vi "DigData.vi"(0 "Type of scan":T14, 1 "Digitizer Settings":T10={"Digitizer delay (us) "=0.0, "rf points per line"=2048, "lines per plane"=128, "Samp Rate (Hz)"=100000000.0, "Additional dig delay (us)"=0.0, "Voltage Scale"=0.4, "Pre-Looks"=0, "Offset delay (us)"=0.0, "bits A/D"=8, "Avg Num"=1, "DigTimeOut"=5.0, "Rel Dig Delay"=0.0, "Dig Ch"=0, "LeCroyCluster"={"LeCroy Channels"=[TRUE, FALSE, FALSE, FALSE], "LC read pt offset"=0.0, "Sweep Avg"=FALSE}, "Main Digitizer"=enum."NI Digitizer", "Dig Config"=enum."Single channel", "Digitizer ID Cluster"={"Acqiris/Alazar/SP ID"=[], "NI Instr Handles"=[], "LeCroy VISA"="", "GaGe Handle"={"Handle"=0, "Sample size"=0, "Resolution"=0, "Offset"=0, "Channels"=0, "Boards"=0}, "ATS Ref"="ATS9350", "Acqiris Address"=["PCI::INSTR0"], "ADQRef"=refnum, "adq_cu_ptr"=refnum}, "Trigger Settings"={"Trig Source"=1, "Trig Coupling"=0, "Trig Slope"=0, "Level (mV)"=1500.0}, "Bulk Acq"=FALSE, "Bulk Start Indexes"=[], "Data Ref RF"=refnum, "NI ID/Channel"=[], "Total Dig CH"=1, "Xtra Ann Trig delay (us)"=10.0, "Fix Z Delay?"=FALSE, "One Way Transmission?"=FALSE, "Data Ref Log"=refnum} {"Trigger Settings"."Trig Slope" items=["Positive", "Negative"]; "Trigger Settings"."Level (mV)" format="%.2f"; "Trigger Settings"."Trig Coupling" items=["DC 1 MOhm", "AC 1 MOhm", "DC 50 Ohm", "AC 50 Ohm"]; "Trigger Settings"."Trig Source" items=["Chan 1", "External"]; "Rel Dig Delay" format="%.2f"; "DigTimeOut" format="%.2f"; "Avg Num" min=1; "Offset delay (us)" format="%.2f"; "Additional dig delay (us)" format="%.2f"; "Digitizer delay (us)" format="%.2f"}, 5 "File Name In":string, 7 "Therapy (T)":bool, 8 "Ann Array Params":T3={"Synth Foc?"=FALSE, "Focal Zones"=41, "Switch T/R"=0, "Trans Geometry (mm)"={"Transducer"=0, "Geo Focus"=12.0, "a (radius)"=3.0, "# of rings"=5, "kerf space "=0.1, "Center Freq"=12.0}, "Sub Ap Excite?"=FALSE, "Full Array Scan?"=FALSE, "Xmt/Rcv"={"XMIT"=[TRUE, TRUE, TRUE, TRUE, TRUE], "RCV"=[TRUE, TRUE, TRUE, TRUE, TRUE]}, "PulseSpacing (us)"=0.0, "Xmit Ring"=0, "XMIT CHS"=0, "RCV CHS"=0, "GPU?"=FALSE, "Save TIFF?"=FALSE, "downfactor"=1, "RCV 1CH"=0} {"RCV 1CH" items=["All", "1", "2", "3", "4", "5"]; "Trans Geometry (mm)"."Transducer" items=["6D 12R 40 MHz"=0, "10D 31R 20 MHz"=1, "10D 23R 20 MHz"=2, "6D 23R 40 MHz"=3, "4.5D 10.7R 40 MHz"=4, "9D 23.5R 20 MHz"=5, "9D 25.8R 20MHz"=6, "Enter"=99]; "Switch T/R" min=1 max=5 step=1}, 9 "Motion Settings In":T6={"No Motion?"=FALSE, "Motion System"=enum."NI 735x", "Motion Bd ID"=1, "Motion Profile"="SMAC1", "# Axis"=1, "Reverse Z axis?"=TRUE, "SMAC Axis"=0, "scan pair"=enum."y-(x) scan", "RT fps"=6.0, "Steps per mm"=[1000, 1000, 1000, 1000], "Motor Parameters"={"velocity ct/s"=[10000.0, 10000.0, 10000.0, 50000.0], "accel ct/s^2"=[50000.0, 50000.0, 50000.0, 200000.0]}, "One Way Scan"=FALSE, "Reverse One Way Scan"=FALSE, "Global Position (mm)"=[], "Plane"=0, "Distance between\nscan lines (um)"=0.0, "Distance between\nscan planes (um)"=0.0, "number of scan planes"=1, "Total steps in line"=0, "Xtra plane\ndistance  (um)"=100, "Xtra planes "=1, "Add Axis"=FALSE, "overshoot cts"=200, "BKPT Shift"=0, "Scan Start Time (ms)"=0, "ESP VISA"="GPIB::1::INSTR", "3rd Axis"=1, "GL Ref Out"=refnum, "Galil Address"=""} {"3rd Axis" items=["x", "y", "z", "w"]; "Xtra planes" min=1; "Xtra plane\ndistance  (um)" min=0; "Distance between\nscan planes (um)" format="%.2f"; "Distance between\nscan lines (um)" format="%.2f"; "SMAC Axis" items=["None"=0, "Axis 1"=1, "Axis 2"=2, "Axis 3"=3, "Axis 4"=4, "Axis 5"=5, "Axis 6"=6, "Axis 7"=7, "Axis 8"=8, "Vector Space 1"=17, "Vector Space 2"=18, "Vector Space 3"=19, "Vector Space 4"=20]; "Motion Bd ID" min=1 max=32 step=1}, 10 "recipient":string, 11 "Microscopy Scan Mode":T2(ring)=enum."Overview Scan", 12 "Breath Divide":i32=1) -> (20 "Scan Params":T1={"File Name"="", "Keep?"=FALSE, "Synth Foc?"=FALSE, "Microscopy Scan Mode"=enum."Overview Scan"}, 27 "Error Message":string)   [LabVIEW 2022 SP3]
uses:
  Controls/ScanType2.ctl
  Digitizers/-DigitizerRoutines/DigitizerSettings.ctl
  Digitizers/-DigitizerRoutines/Digitizer.ctl
  Digitizers/-DigitizerRoutines/DigConfig.ctl
  Digitizers/-DigitizerRoutines/DigitizerID.ctl
  C:/Windows/System32/ADQAPI_dotNet_helper.dll
  Windows/System32/ADQAPI_dotNet_helper.dll
  Motion Controllers/NI_controller/-NI_MotionRoutines/MotionParameters.ctl
  Motion Controllers/NI_controller/-NI_MotionRoutines/MotionSys.ctl
  Motion Controllers/-MotionRoutines/ScanAxis.ctl
  Motion Controllers/-MotionRoutines/3rdAxis.ctl
  Annular Array/-AnnularRoutines/AnnularArray.ctl
  Annular Array/-AnnularRoutines/TransGeometry.ctl
  Annular Array/-AnnularRoutines/ArrayGeometry.ctl
  Controls/ScanParams.ctl
  Motion Controllers/Galil/Command Menu.ctl
  <vilib>/DAQmx/write.llb/DAQmx Write (Digital Bool 1Line 1Point).vi
  Motion Controllers/-MotionRoutines/MotionGlobals.vi
  Pulsers/PulserGlobals.vi
  <vilib>/DAQmx/create/channels.llb/DAQmx Create Channel (CO-Pulse Generation-Frequency).vi
  <vilib>/DAQmx/configure/timing.llb/DAQmx Timing (Implicit).vi
  <vilib>/DAQmx/miscellaneous.llb/DAQmx Fill In Error Info.vi
  <vilib>/DAQmx/create/channels.llb/DAQmx Create Channel (AI-Voltage-Basic).vi
  <vilib>/DAQmx/configure/timing.llb/DAQmx Timing (Sample Clock).vi
  <vilib>/DAQmx/configure/trigger.llb/DAQmx Start Trigger (Digital Edge).vi
  Switch Modules/SwitchGlobals.vi
  Motion Controllers/Galil/GL Axis Control.ctl
  <vilib>/Utility/SMTP/NI_SMTPEmail.lvlib
  <vilib>/Motion/FlexMotion/CustomControls/CustomControls.llb/Mask (8 axes).flx
  <vilib>/Motion/FlexMotion/FunctionsVIs/Trajectory.llb/Load Acceleration/Deceleration.flx
  <instrlib>/Newport ESP301/Newport ESP301.lvlib
  <instrlib>/LeCroy Wave Series/LeCroy Wave Series.lvlib
  <vilib>/Motion/FlexMotion/FunctionsVIs/MotionIO.llb/Set Inhibit MOMO (8 axes).flx
panel:
  out "x-y":u32
  out "Current Plane":i32
  # "First axis used in 1-D\nscan"
  # "1-D and 2-D B scan settings"
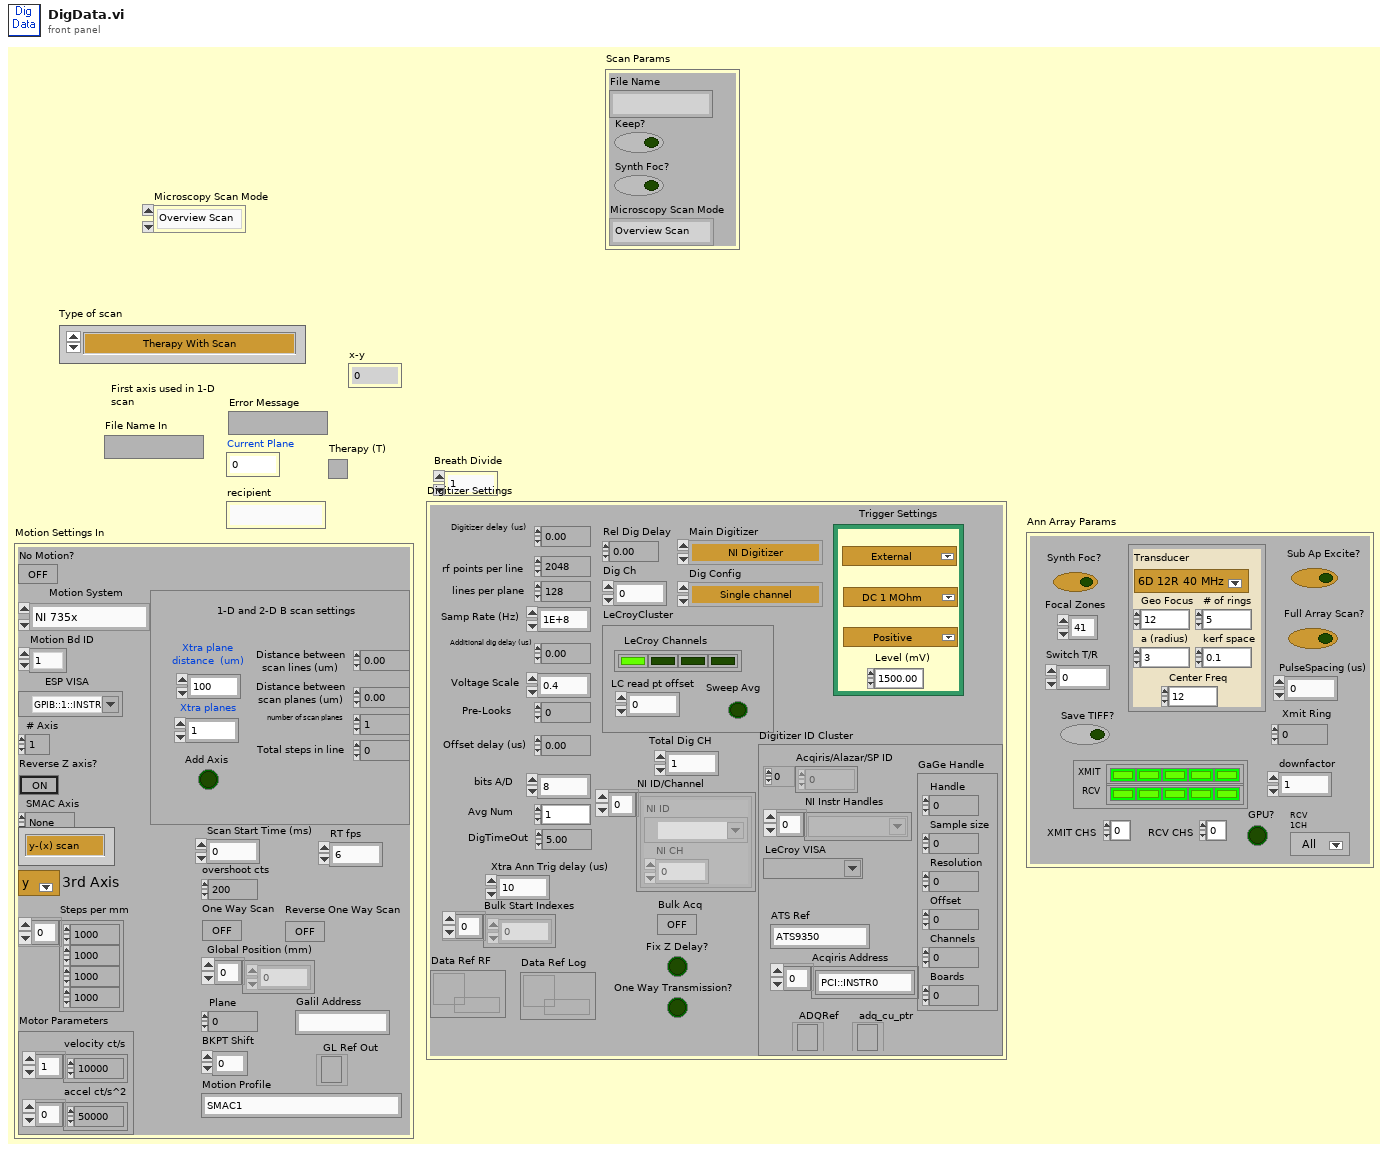
[diagram p1: front panel]
types:
  T1 = typedef "ScanParams.ctl" = cluster{"File Name":string, "Keep?":bool, "Synth Foc?":bool, "Microscopy Scan Mode":enum32{"Level X", "Level Y", "Overview Scan", "Detailed Scan", "V-Z Scan"}}
  T2 = enum32{"Level X", "Level Y", "Overview Scan", "Detailed Scan", "V-Z Scan"}
  T3 = typedef "AnnularArray.ctl" = cluster{"Synth Foc?":bool, "Focal Zones":i16, "Switch T/R":i16, "Trans Geometry (mm)":T4, "Sub Ap Excite?":bool, "Full Array Scan?":bool, "Xmt/Rcv":cluster{"XMIT":bool[], "RCV":bool[]}, "PulseSpacing (us)":sgl, "Xmit Ring":i32, "XMIT CHS":u8, "RCV CHS":u8, "GPU?":bool, "Save TIFF?":bool, "downfactor":i32, "RCV 1CH":u16}
  T4 = typedef "TransGeometry.ctl" = cluster{"Transducer":T5, "Geo Focus":dbl, "a (radius)":dbl, "# of rings":i32, "kerf space ":dbl, "Center Freq":dbl}
  T5 = typedef "ArrayGeometry.ctl" = u16
  T6 = typedef "MotionParameters.ctl" = cluster{"No Motion?":bool, "Motion System":T7, "Motion Bd ID":u8, "Motion Profile":string, "# Axis":i8, "Reverse Z axis?":bool, "SMAC Axis":u16, "scan pair":T8, "RT fps":sgl, "Steps per mm":i32[], "Motor Parameters":cluster{"velocity ct/s":dbl[], "accel ct/s^2":dbl[]}, "One Way Scan":bool, "Reverse One Way Scan":bool, "Global Position (mm)":dbl[], "Plane":i32, "Distance between\nscan lines (um)":sgl, "Distance between\nscan planes (um)":sgl, "number of scan planes":i32, "Total steps in line":i32, "Xtra plane\ndistance  (um)":i32, "Xtra planes ":i32, "Add Axis":bool, "overshoot cts":i32, "BKPT Shift":i32, "Scan Start Time (ms)":u32, "ESP VISA":refnum<visa-resource-name>, "3rd Axis":T9, "GL Ref Out":refnum<k7>, "Galil Address":string}
  T7 = typedef "MotionSys.ctl" = enum16{"MM3000", "NI 735x", "Newport ESP", "No Motion Card", "Galil"}
  T8 = typedef "ScanAxis.ctl" = enum16{"y-(x) scan", "x-(y) scan", "z-(x) scan", "z-(y) scan", "y-(z) scan", "x-(z) scan", "w-(x) scan", "w-(y) scan", "w-(z) scan", "x-(w) scan", "y-(w) scan", "z-(w) scan"}
  T9 = typedef "3rdAxis.ctl" = u16
  T10 = typedef "DigitizerSettings.ctl" = cluster{"Digitizer delay (us) ":dbl, "rf points per line":i32, "lines per plane":i32, "Samp Rate (Hz)":dbl, "Additional dig delay (us)":dbl, "Voltage Scale":dbl, "Pre-Looks":i32, "Offset delay (us)":dbl, "bits A/D":i8, "Avg Num":i32, "DigTimeOut":sgl, "Rel Dig Delay":sgl, "Dig Ch":i32, "LeCroyCluster":cluster{"LeCroy Channels":bool[], "LC read pt offset":dbl, "Sweep Avg":bool}, "Main Digitizer":T11, "Dig Config":T12, "Digitizer ID Cluster":T13, "Trigger Settings":cluster{"Trig Source":u16, "Trig Coupling":u16, "Trig Slope":u16, "Level (mV)":dbl}, "Bulk Acq":bool, "Bulk Start Indexes":i32[], "Data Ref RF":refnum<data-value>, "NI ID/Channel":cluster{"NI ID":refnum<k15>, "NI CH":i32}[], "Total Dig CH":i32, "Xtra Ann Trig delay (us)":dbl, "Fix Z Delay?":bool, "One Way Transmission?":bool, "Data Ref Log":refnum<data-value>}
  T11 = typedef "Digitizer.ctl" = enum16{"Acqiris Digitizer", "NI Digitizer", "LeCroy", "GaGe", "AlazarTech", "No Digitizer", "Teledyne"}
  T12 = typedef "DigConfig.ctl" = enum16{"Single channel", "2 Chans w/ 2 Acqiris", "2 Chans w/ 1 Acqiris", "5-CH Pulser New", "5-CH pulser w/ ann array", "5-pass style ann array", "Empty"}
  T13 = typedef "DigitizerID.ctl" = cluster{"Acqiris/Alazar/SP ID":u32[], "NI Instr Handles":refnum<k15>[], "LeCroy VISA":refnum<visa-resource-name>, "GaGe Handle":cluster{"Handle":u32, "Sample size":u32, "Resolution":i32, "Offset":i32, "Channels":u32, "Boards":u32}, "ATS Ref":string, "Acqiris Address":string[], "ADQRef":refnum<k24>, "adq_cu_ptr":refnum<k24>}
  T14 = typedef "ScanType2.ctl" = enum16{"Therapy With Scan", "M scan", "M Scan With Therapy Burst", "1-D B Scan", "1-D B Scan With Therapy Burst", "2-D B Scan", "2-D B Scan With Therapy Burst", "Rotational Scan", "1-D B-Scan PRF", "2-D B-Scan PRF", "Real-Time Scan", "Contrast Agents", "1-D w/ Real-Time Set Up", "Dual Transducer", "Acoustic Microscopy", "Hydrophone Scanning"}
  T15 = typedef "EKG_Mode.ctl" = u16
  T16 = typedef "Mask (8 axes).flx" = cluster{"1":bool, "2":bool, "3":bool, "4":bool, "5":bool, "6":bool, "7":bool, "8":bool}
  T17 = typedef "Command Menu.ctl" = enum16{"CommandPassThrough", "Abort Motion", "Define Pos", "Velocity", "Acceleration", "Deceleration", "Position Rel", "Postion Abs", "Begin Move", "After Move", "Home", "KI", "KD", "KP", "IL", "Config I/O", "Set Bit", "Clear Bit", "Motor Off", "Moto On", "Status", "Execute", "Halt Execute", "HX Status", "Tell Velocity", "Check Motion", "BreakPoint", "Tell Position", "Current Code Line", "Tell Switches", "OC Force On", "OC Off", "Pos Soft Limit", "Rev Soft Limit"}
  T18 = enum16{"Absolute Position", "Relative Position", "Velocity", "Relative to Cap Pos", "Modulus Position", "Absolute Contouring", "Relative Contouring"}
  T19 = typedef "GL Axis Control.ctl" = u16
  T20 = typedef "pulser.ctl" = enum16{"Pan 5900", "Daxsonics", "Agilent 33xxx", "UTEX", "JSR", "WMC Mono-Cycle", "No Pulser", "NYU AVTECH", "Tabor W1281A", "Pan 5800", "Unlisted", "Tabor WX2182B"}
  T21 = cluster{"Energy (microJ)":u8, "Damping (In Ohm)":u8, "HP Filt(KHz) ":u8, "LP Filt (MHz)":u8, "Gain (db)":u8, "Atten (dB)":sgl}
  T22 = typedef "Resource Out (Enum).flx" = u16
  T23 = typedef "SwitchOption.ctl" = enum16{"Cytex", "Pickering", "NI Switch", "No Switch", "Riverside USB"}
  T24 = typedef "Breath_Mode.ctl" = u16
  T25 = cluster{sgl, "Gain [dB]  ":sgl, "Atten (dB)":sgl}
  T26 = typedef "Bd Id Out" = u8
  T27 = cluster{"File Name In":string, bool, "Synth Foc?":bool, "Microscopy Scan Mode":enum32{"Level X", "Level Y", "Overview Scan", "Detailed Scan", "V-Z Scan"}}
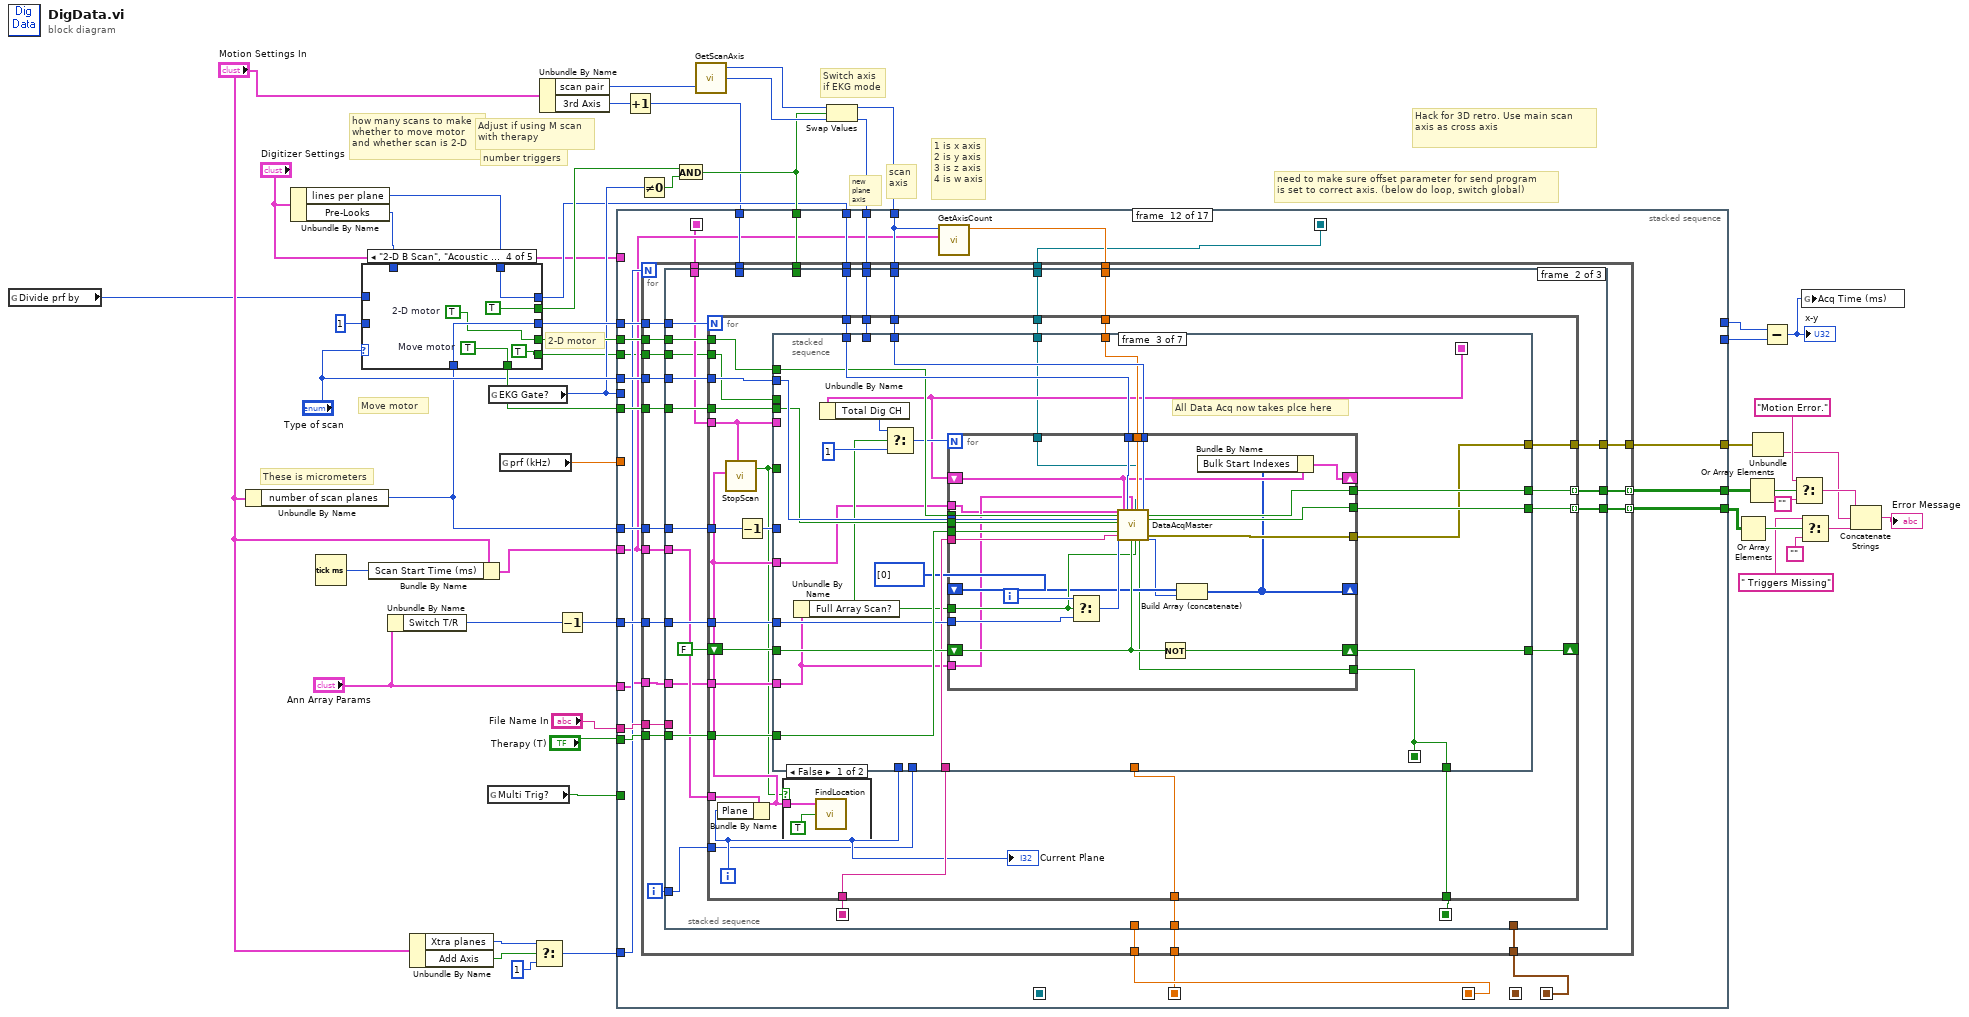
[diagram p0: block diagram]
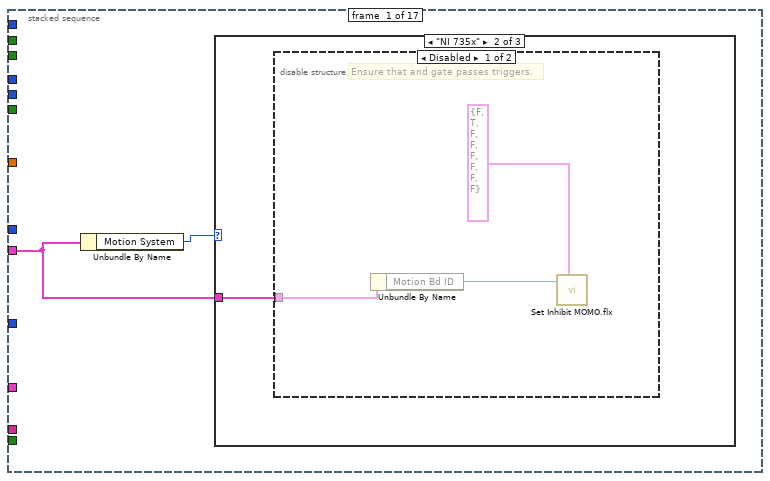
[diagram p2: hidden frame]
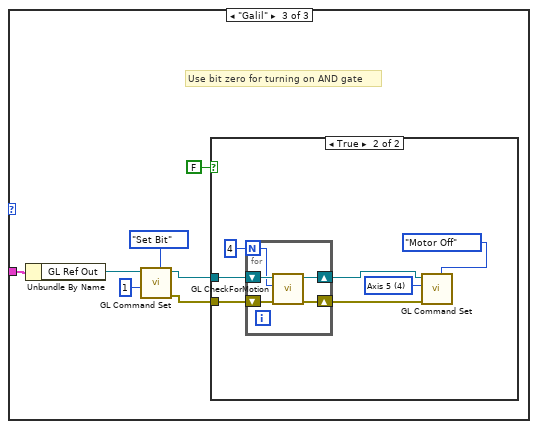
[diagram p5: hidden frame]
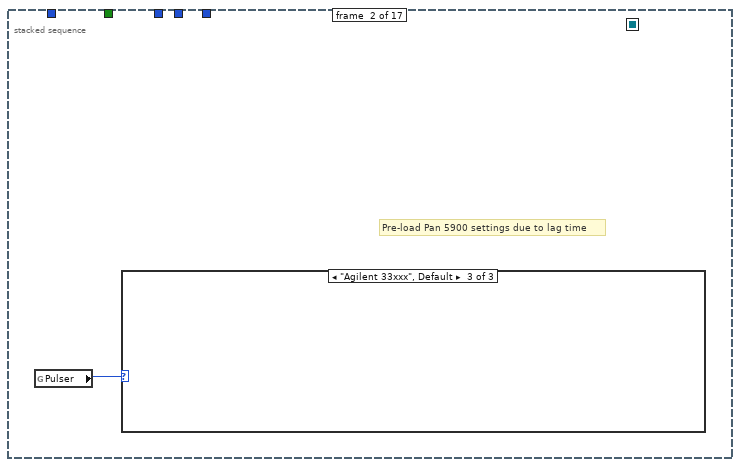
[diagram p7: hidden frame]
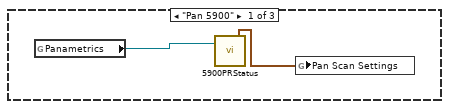
[diagram p8: hidden frame]
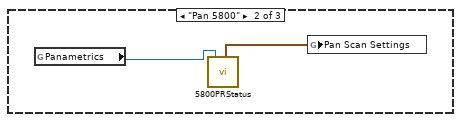
[diagram p9: hidden frame]
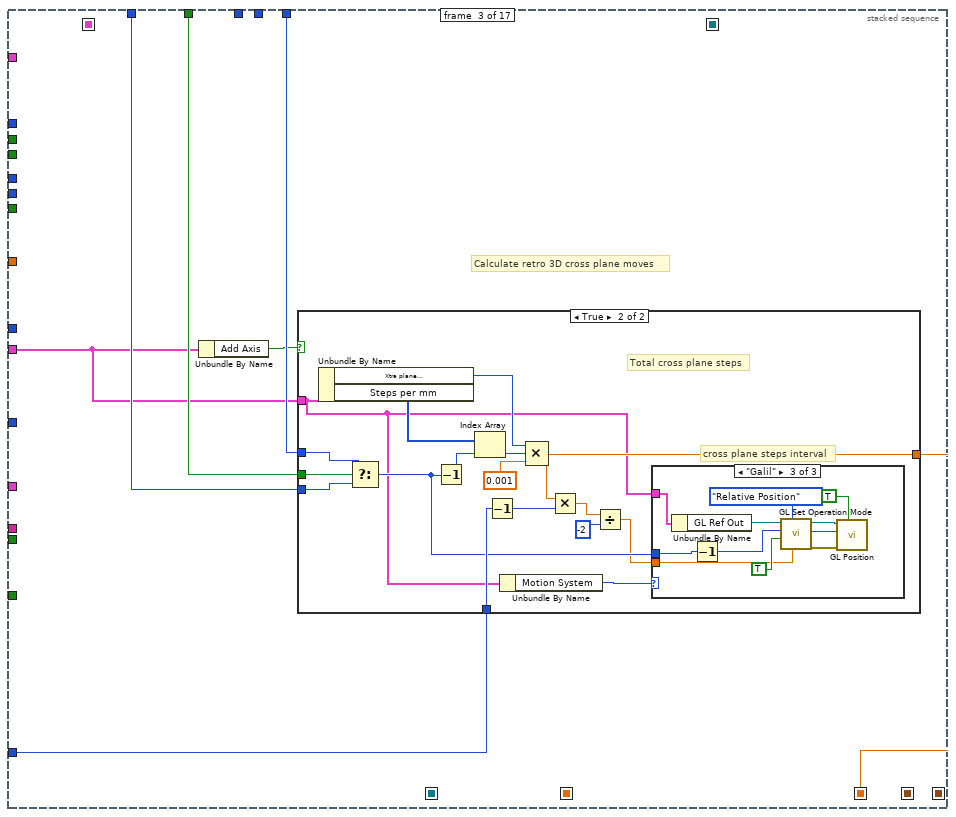
[diagram p10: hidden frame]
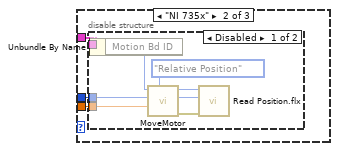
[diagram p13: hidden frame]
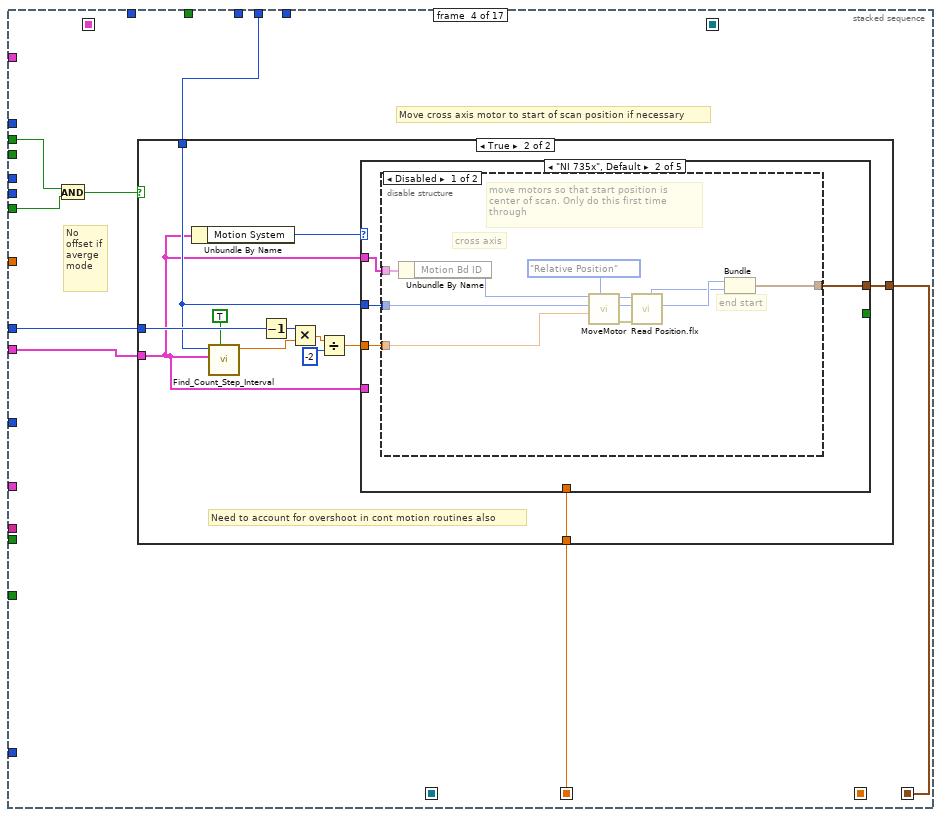
[diagram p15: hidden frame]
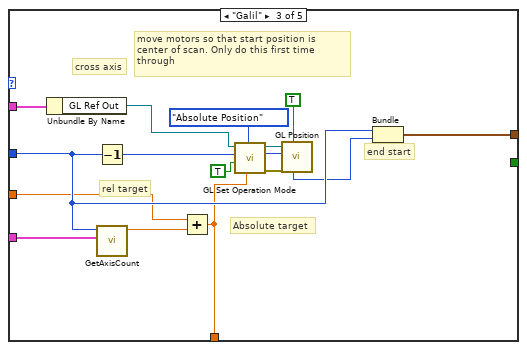
[diagram p19: hidden frame]
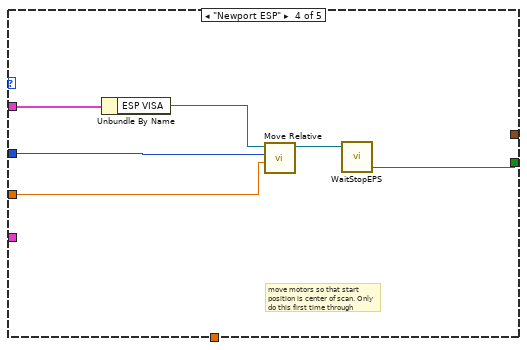
[diagram p20: hidden frame]
diagram:
  # "Move motor"
  # "2-D motor"
  # "Hack for 3D retro. Use main scan axis as cross axis"
  # "Switch axis if EKG mode"
  # "new plane axis"
  # "scan axis"
  # "1 is x axis\n2 is y axis\n3 is z axis\n4 is w axis"
  # "need to make sure offset parameter for send program\nis set to correct axis. (below do loop, switch global)"
  # "Adjust if using M scan\nwith therapy"
  # "These is micrometers"
  # "number triggers"
  # "how many scans to make\nwhether to move motor\nand whether scan is 2-D"
  n1 = global read "PulserGlobals.vi" "Divide prf by"() -> (w7:i32)
  n2 = Unbundle By Name("Motion Settings In") -> ("number of scan planes"=w13:i32)
  n3 = Unbundle By Name("Digitizer Settings") -> ("lines per plane"=w18:i32, "Pre-Looks"=w17:i32)
  n4 = Tick Count (ms)() -> (millisecond timer value=w9:u32)
  n5 = case shown="\"2-D B Scan\", \"Acoustic Microscopy\"" "Type of scan" {
    tunnel: [w56 w65 w69 w75 w80] -> w38
    tunnel: 1 -> [w56 w65 w69 _ _]
    tunnel: w13 -> [_ _ _ w75 w80]
    tunnel: [_ _ w67 w71 w77] -> w52
    tunnel: [_ _ _ w72 w78] -> w51
    tunnel: [w55 w63 w68 w74 w79] -> w22
    tunnel: w18 -> [w55 w60 w68 w74 w79]
    tunnel: w7 -> [_ w59 _ _ _]
    tunnel: w17 -> [_ w58 _ _ _]
    tunnel: [_ _ _ TRUE _] -> w25
    tunnel: [FALSE FALSE FALSE TRUE TRUE] -> w2
    frame "Therapy With Scan", Default {
    }
    frame "M Scan With Therapy Burst" {
      n6 = Less?(x=w59, y=w58) -> (x < y?=w64:bool)
      n7 = Subtract(x=w59, y=w58) -> (x-y=w62:i32)
      n8 = Add(x=w60, y=w62) -> (x+y=w61:i32)
      n9 = Select(t=w60, s=w64, f=w61) -> (s? t:f=w63:i32)
    }
    frame "1-D B Scan", "1-D B Scan With Therapy Burst", "1-D B-Scan PRF", "1-D w/ Real-Time Set Up" {
      w67 = TRUE  # Move motor
    }
    frame "2-D B Scan", "Acoustic Microscopy" {
      w71 = TRUE  # Move motor
      w72 = TRUE  # 2-D motor
    }
    frame "2-D B Scan With Therapy Burst", "Rotational Scan", "2-D B-Scan PRF" {
      w77 = TRUE  # Move motor
      w78 = TRUE  # 2-D motor
    }
  }
  n10 = Bundle By Name(cluster="Motion Settings In", "Scan Start Time (ms)"=w9) -> (w10:T6)
  n11 = Unbundle By Name("Ann Array Params") -> ("Switch T/R"=w5:i16)
  n12 = Unbundle By Name("Motion Settings In") -> ("Xtra planes"=w12:i32, "Add Axis"=w15:bool)
  n13 = global read "MotionGlobals.vi" "Multi Trig?"() -> (w29:bool)
  n14 = global read "MotionGlobals.vi" "EKG Gate?"() -> (w24:T15)
  n15 = global read "PulserGlobals.vi" "prf (kHz)"() -> (w8:dbl)
  n16 = Select(t=w12, s=w15, f=1) -> (s? t:f=w19:i32)
  n17 = Unbundle By Name("Motion Settings In") -> ("scan pair"=w14:T8, "3rd Axis"=w4:T9)
  n18 = Decrement(x=w5) -> (x-1=w36:i16)
  n19 = Increment(x=w4) -> (x+1=w3:T9)
  n20 = Not Equal To 0?(x=w24) -> (x != 0?=w26:bool)
  n21 = And(x=w25, y=w26) -> (x .and. y?=w23:bool)
  n22 = call "GetScanAxis.vi"("scan pair"=w14) -> ("Axis 1"=w28:i32, "Axis 2"=w27:i32)  [unwired: 1 in, 1 out]
  n23 = Swap Values(12:w28, 13:w23, 14:w27) -> (1:w16:i32, 3:w21:i32)
  n24 = stacked-sequence {
    seq-local: [_ _ _ _ _ _ _ _ w331 _ _ _ _ _ _ _ _] -> [_ _ _ _ _ _ _ _ _ _ _ w408 _ _ _ w954 _]
    seq-local: [_ _ _ _ _ _ _ w274 _ _ _ _ _ _ _ _ _] -> [_ _ _ _ _ _ _ _ _ _ _ _ _ _ _ w953 _]
    seq-local: [_ _ w113 _ _ _ _ _ _ _ _ _ _ _ _ _ _] -> [_ _ _ _ _ _ _ _ _ _ _ w419 _ _ _ _ _]
    seq-local: [_ _ _ w162 _ _ _ _ _ _ _ _ _ _ _ _ _] -> [_ _ _ _ w220 _ _ _ _ _ _ _ _ _ _ _ _]
    seq-local: [_ _ _ _ w218 _ _ _ _ _ _ _ _ _ _ _ _] -> [_ _ _ _ _ _ _ _ _ _ _ w414 _ _ _ _ _]
    seq-local: [_ _ _ _ _ _ _ _ _ _ w379 _ _ _ _ _ _] -> [_ _ _ _ _ _ _ _ _ _ _ w412 _ _ _ w949 _]
    seq-local: [_ _ _ w157 _ _ _ _ _ _ _ _ _ _ _ _ _] -> [_ _ _ _ _ _ _ _ _ _ _ w409 _ _ _ _ _]
    tunnel: w52 -> [_ _ _ w161 w216 _ _ w276 _ _ _ w433 _ w891 _ _ w960]
    tunnel: w51 -> [_ _ _ w160 _ _ _ _ _ _ w378 w432 _ _ w937 _ _]
    tunnel: "Therapy (T)" -> [_ _ _ _ _ _ _ _ _ _ _ w431 _ _ _ _ _]
    tunnel: [_ _ _ _ _ _ _ _ _ _ _ w430 _ _ _ _ _] -> w37
    tunnel: w22 -> [_ _ _ _ _ _ _ _ w334 _ w382 w429 _ _ _ _ _]
    tunnel: w21 -> [_ _ _ w164 _ _ _ _ _ _ _ w428 _ _ _ _ _]
    tunnel: w16 -> [_ _ w116 _ w222 _ _ w275 _ _ _ w416 w838 _ _ _ _]
    tunnel: [_ _ _ _ _ _ _ _ _ _ _ w427 _ _ _ _ _] -> w43
    tunnel: "Type of scan" -> [_ _ _ _ _ _ _ _ _ _ _ w426 _ _ _ _ _]
    tunnel: w38 -> [_ _ _ _ _ _ _ _ _ _ _ w425 _ _ _ _ _]
    tunnel: w13 -> [_ _ _ w163 _ _ _ _ _ _ _ w423 _ _ _ _ _]
    tunnel: w36 -> [_ _ _ _ _ _ _ _ _ _ _ w424 _ _ _ _ _]
    tunnel: "File Name In" -> [_ _ _ _ _ _ _ _ _ _ _ w422 _ _ w939 _ _]
    tunnel: [_ _ _ _ _ _ _ _ _ _ _ w421 _ _ _ _ _] -> w34
    tunnel: w24 -> [_ _ _ _ w225 _ w257 _ w332 _ _ _ _ _ _ w955 _]
    tunnel: [_ _ _ _ _ _ w256 _ _ _ _ _ _ _ _ _ _] -> w31
    tunnel: [_ _ _ _ _ _ _ _ _ _ _ _ w833 _ _ _ _] -> w32
    tunnel: w29 -> [_ _ _ _ _ _ w255 _ _ _ _ _ _ _ _ _ _]
    tunnel: w23 -> [_ _ w115 _ w221 _ _ _ _ _ _ w418 _ _ _ _ _]
    tunnel: w8 -> [_ _ _ _ _ _ w254 _ w333 _ _ _ _ _ _ _ _]
    tunnel: w19 -> [_ _ w117 _ _ _ _ _ _ _ _ w420 _ _ _ _ _]
    tunnel: w3 -> [_ _ w114 _ _ _ _ _ _ _ _ w417 _ _ _ _ _]
    tunnel: "Digitizer Settings" -> [_ _ _ _ w215 _ w253 w273 _ _ w381 _ _ _ _ _ _]
    tunnel: w10 -> [w81 _ w111 w158 w214 w239 _ w271 _ _ _ w413 w834 w892 _ _ w961]
    tunnel: "Ann Array Params" -> [_ _ _ _ _ _ _ w270 _ w371 w376 w411 _ _ w936 _ _]
    tunnel: w2 -> [_ _ _ _ _ _ _ _ _ _ _ w410 _ _ _ _ _]
    frame #0 {
      n25 = Unbundle By Name(w81) -> ("Motion System"=w82:T7)
      n26 = case shown="\"NI 735x\"" w82 {
        tunnel: w81 -> [_ w83 w93]
        frame "No Motion Card", Default {
        }
        frame "NI 735x" {
          n27 = disable-structure shown="Disabled" {
            disable-tunnel: w83 -> [w85 _]
            frame Disabled {
              # "Ensure that and gate passes triggers."
              n28 = Unbundle By Name(w85) -> ("Motion Bd ID"=w84:u8)
              n29 = call-poly <vilib>:"Set Inhibit MOMO.flx"("Must On (False)"=T16 {"1"=FALSE, "2"=TRUE, "3"=FALSE, "4"=FALSE, "5"=FALSE, "6"=FALSE, "7"=FALSE, "8"=FALSE}, "Board ID"=w84) -> ()  [unwired: 2 in, 6 out]
            }
            frame Enabled {
            }
          }
        }
        frame "Galil" {
          # "Use bit zero for turning on AND gate"
          n30 = Unbundle By Name(w93) -> ("GL Ref Out"=w92:refnum<k7>)
          n31 = call "GL Command Set.vi"("Command"=Command_Menu."Set Bit", "Value"=1, "Galil.IGalil"=w92) -> ("error out"=w88:errorcluster, "ref out"=w89:refnum<k7>)  [unwired: 4 in, 3 out]
          n32 = case shown="True" FALSE {
            tunnel: w89 -> [_ w98]
            tunnel: w88 -> [_ w97]
            frame False {
            }
            frame True {
              w100 = T19 4 items=["Axis 1", "Axis 2", "Axis 3", "Axis 4", "Axis 5", "Axis 6", "Axis 7", "Axis 8"] ("Axis")
              n33 = for {
                N: 4 -> [w101]
                shift-right: [w102] -> w95
                shift-left: w98 -> [w105]
                shift-right: [w103] -> w96
                shift-left: w97 -> [w104]
                n34 = call "GL CheckForMotion.vi"("error in"=w104, "Axis"=w101, "Refnum in"=w105) -> ("error out"=w103:errorcluster, "Refnum out"=w102:refnum<k7>)  [unwired: 6 in, 1 out]
              }
              n35 = call "GL Command Set.vi"("Command"=Command_Menu."Motor Off", "error in (no error)"=w96, "Axis"=w100, "Galil.IGalil"=w95) -> ()  [unwired: 3 in, 5 out]
            }
          }
        }
      }
    }
    frame #1 {
      # "Pre-load Pan 5900 settings due to lag time"
      n36 = global read "PulserGlobals.vi" "Pulser"() -> (w106:T20)
      n37 = case shown="\"Agilent 33xxx\", Default" w106 {
        frame "Pan 5900" {
          n38 = global read "PulserGlobals.vi" "Panametrics"() -> (w107:refnum<visa-resource-name>)
          n39 = call "5900PRStatus.vi"("VISA resource name"=w107) -> ("Pan Scan Settings"=w108:T21)  [unwired: 1 in, 3 out]
          n40 = global write "PulserGlobals.vi" "Pan Scan Settings"(w108) -> ()
        }
        frame "Pan 5800" {
          n41 = global read "PulserGlobals.vi" "Panametrics"() -> (w109:refnum<visa-resource-name>)
          n42 = call "5800PRStatus.vi"("VISA resource name"=w109) -> ("Pan Scan Settings"=w110:T21)  [unwired: 8 in, 10 out]
          n43 = global write "PulserGlobals.vi" "Pan Scan Settings"(w110) -> ()
        }
        frame "Agilent 33xxx", Default {
        }
      }
    }
    frame #2 {
      # "Calculate retro 3D cross plane moves"
      n44 = Unbundle By Name(w111) -> ("Add Axis"=w112:bool)
      n45 = case shown="True" w112 {
        tunnel: w117 -> [_ w130]
        tunnel: w116 -> [_ w127]
        tunnel: [_ w129] -> w113
        tunnel: w115 -> [_ w128]
        tunnel: w114 -> [_ w126]
        tunnel: w111 -> [_ w118]
        frame False {
        }
        frame True {
          # "cross plane steps interval"
          # "Total cross plane steps"
          n46 = Unbundle By Name(w118) -> ("Xtra plane\ndistance  (um)"=w121:i32, "Steps per mm"=w120:i32[])
          n47 = Select(t=w127, s=w128, f=w126) -> (s? t:f=w123:i32)
          n48 = Decrement(x=w123) -> (x-1=w133:i32)
          n49 = Index Array(array=w120, index=w133) -> (element=w134:i32)
          n50 = Decrement(x=w130) -> (x-1=w131:i32)
          n51 = Unbundle By Name(w118) -> ("Motion System"=w119:T7)
          n52 = Compound Arithmetic op=MULTIPLY(w121, w134, 0.001) -> (w129:dbl)
          n53 = Multiply(x=w129, y=w131) -> (x*y=w124:dbl)
          n54 = Divide(x=w124, y=-2) -> (x/y=w122:dbl)
          n55 = case shown="\"Galil\"" w119 {
            tunnel: w123 -> [_ w137 w153]
            tunnel: w122 -> [_ w136 w150]
            tunnel: w118 -> [_ w135 w155]
            frame "MM3000", Default {
            }
            frame "NI 735x" {
              n56 = disable-structure shown="Disabled" {
                disable-tunnel: w137 -> [w145 _]
                disable-tunnel: w136 -> [w142 _]
                disable-tunnel: w135 -> [w139 _]
                frame Disabled {
                  n57 = Unbundle By Name(w139) -> ("Motion Bd ID"=w138:u8)
                  n58 = call "MoveMotor.vi"("Position Mode (Absolute)"=T18."Relative Position", "Target Position (0)"=w142, "Axis or Vector Space"=w145, "Motion Bd ID"=w138) -> ("error out"=w143:errorcluster, "Resource Output"=w140:u16, "Bd ID Out"=w141:u8)  [unwired: 5 in]
                  n59 = call <vilib>:"Read Position.flx"("error in (no error)"=w143, "Axis"=w140, "Board ID"=w141) -> ()  [unwired: 3 in, 4 out]
                }
                frame Enabled {
                }
              }
            }
            frame "Galil" {
              n60 = Unbundle By Name(w155) -> ("GL Ref Out"=w154:refnum<k7>)
              n61 = Decrement(x=w153) -> (x-1=w152:i32)
              n62 = call "GL Set Operation Mode.vi"("position cts (abs/rel)"=w150, "Position Mode (Absolute)"=T18."Relative Position", "Start Now?"=TRUE, "Axis"=w152, "Galil.IGalil"=w154) -> ("error out"=w148:errorcluster, "Axis Out Output"=w147:T19, "Galil Out"=w149:refnum<k7>)  [unwired: 4 in]
              n63 = call "GL Position.vi"("Wait for Motion Complete"=TRUE, "error in (no error)"=w148, "Axis"=w147, "Galil.IGalil"=w149) -> ()  [unwired: 2 in, 4 out]
            }
          }
        }
      }
    }
    frame #3 {
      # "No offset if averge mode"
      # "Move cross axis motor to start of scan position if necessary"
      n64 = And(x=w160, y=w161) -> (x .and. y?=w159:bool)
      n65 = case shown="True" w159 {
        tunnel: w164 -> [_ w169]
        tunnel: w163 -> [_ w172]
        tunnel: [_ w176] -> w162
        tunnel: w158 -> [_ w166]
        tunnel: [_ w165] -> w157
        frame False {
          # "Can use this option if don't want start point to be center of scan."
        }
        frame True {
          # "Need to account for overshoot in cont motion routines also"
          n66 = Unbundle By Name(w166) -> ("Motion System"=w170:T7)
          n67 = call "Find_Count_Step_Interval.vi"("BP Int (F)/Plane Int (T)"=TRUE, "Motion Settings In"=w166, "Axis"=w169) -> ("BP Interval"=w168:dbl)  [unwired: 7 in, 1 out]
          n68 = Decrement(x=w172) -> (x-1=w174:i32)
          n69 = Multiply(x=w174, y=w168) -> (x*y=w173:dbl)
          n70 = Divide(x=w173, y=-2) -> (x/y=w171:dbl)
          n71 = case shown="\"NI 735x\", Default" w170 {
            tunnel: w169 -> [_ w180 w196 w213 _]
            tunnel: [_ w179 w207 _ _] -> w176
            tunnel: [_ _ _ w211 _] -> _
            tunnel: w171 -> [_ w178 w194 w210 _]
            tunnel: w166 -> [_ w177 w205 w209 _]
            tunnel: w166 -> [_ _ w197 _ _]
            tunnel: [_ _ w193 _ _] -> w165
            frame "MM3000" {
            }
            frame "NI 735x", Default {
              n72 = disable-structure shown="Disabled" {
                disable-tunnel: w180 -> [w191 _]
                disable-tunnel: [w190 _] -> w179
                disable-tunnel: w178 -> [w184 _]
                disable-tunnel: w177 -> [w182 _]
                frame Disabled {
                  # "end start"
                  # "cross axis"
                  # "move motors so that start position is center of scan. Only do this first time through"
                  n73 = Unbundle By Name(w182) -> ("Motion Bd ID"=w181:u8)
                  n74 = call "MoveMotor.vi"("Position Mode (Absolute)"=T18."Relative Position", "Target Position (0)"=w184, "Axis or Vector Space"=w191, "Motion Bd ID"=w181) -> ("error out"=w187:errorcluster, "Resource Output"=w185:u16, "Bd ID Out"=w186:u8)  [unwired: 5 in]
                  n75 = call <vilib>:"Read Position.flx"("error in (no error)"=w187, "Axis"=w185, "Board ID"=w186) -> ("Resource Output"=w189:T22, "Position"=w188:i32)  [unwired: 3 in, 2 out]
                  n76 = Bundle("Resource Output"=w189, "Position"=w188) -> (w190:cluster{"Resource Output":T22, "Position":i32})  [unwired: 1 in]
                }
                frame Enabled {
                }
              }
            }
            frame "Galil" {
              # "rel target"
              # "Absolute target"
              # "end start"
              # "cross axis"
              # "move motors so that start position is center of scan. Only do this first time through"
              n77 = Unbundle By Name(w205) -> ("GL Ref Out"=w203:refnum<k7>)
              n78 = Decrement(x=w196) -> (x-1=w198:i32)
              n79 = call "GetAxisCount.vi"("Motion Settings"=w197, "Scan Axis"=w196) -> ("Counts"=w195:dbl)  [unwired: 9 in]
              n80 = Add(x=w194, y=w195) -> (x+y=w193:dbl)
              n81 = call "GL Set Operation Mode.vi"("position cts (abs/rel)"=w193, "Position Mode (Absolute)"=T18."Absolute Position", "Start Now?"=TRUE, "Axis"=w198, "Galil.IGalil"=w203) -> ("error out"=w200:errorcluster, "Axis Out Output"=w199:T19, "Galil Out"=w202:refnum<k7>)  [unwired: 4 in]
              n82 = call "GL Position.vi"("Wait for Motion Complete"=TRUE, "error in (no error)"=w200, "Axis"=w199, "Galil.IGalil"=w202) -> ("Axis Position"=w192:i32)  [unwired: 2 in, 3 out]
              n83 = Bundle(w196, "Axis Position"=w192) -> (w207:cluster{i32, "Axis Position":i32})  [unwired: 1 in]
            }
            frame "Newport ESP" {
              # "move motors so that start position is center of scan. Only do this first time through"
              n84 = Unbundle By Name(w209) -> ("ESP VISA"=w208:refnum<visa-resource-name>)
              n85 = call <instrlib>:"Move Relative.vi"("Position (0 units)"=w210, "Axis (1)"=w213, "VISA resource name"=w208) -> ("VISA resource name out"=w212:refnum<visa-resource-name>)  [unwired: 3 in, 1 out]
              n86 = call "WaitStopEPS.vi"("VISA resource name"=w212) -> ("Error Status"=w211:bool)  [unwired: 2 in, 2 out]
            }
            frame "No Motion Card" {
            }
          }
        }
      }
    }
    frame #4 {
      # "Get motor ready for scan. Can set to start 1/2 way back in motion"
      # "Skip loading motion program if no motion\nor EKG gate mode."
      # "No scan direction if retro mode."
      n87 = Not(x=w216) -> (.not. x?=w223:bool)
      n88 = Not Equal To 0?(x=w225) -> (x != 0?=w224:bool)
      n89 = Or(x=w224, y=w223) -> (x .or. y?=w217:bool)
      n90 = case shown="True" w216 {
        tunnel: w215 -> [_ w231]
        tunnel: w222 -> [_ w230]
        tunnel: w221 -> [_ w229]
        tunnel: [_ w228] -> w219
        tunnel: w217 -> [_ w227]
        tunnel: w214 -> [_ w226]
        frame False {
        }
        frame True {
          n91 = case shown="False" w227 {
            tunnel: w231 -> [w232 _]
            tunnel: w230 -> [w234 _]
            tunnel: w229 -> [w237 _]
            tunnel: [w235 _] -> w228
            tunnel: w226 -> [w233 _]
            frame False {
              n92 = Not(x=w237) -> (.not. x?=w236:bool)
              n93 = call "PrepForScan.vi"("Motion Settings In"=w233, "SMAC?"=FALSE, "Scan Axis"=w234, "MoveBack?"=w236, "Digitizer Settings"=w232) -> ("Axis Move Info"=w235:cluster{"Resource Output":u16, "Position":i32})  [unwired: 5 in, 5 out]
            }
            frame True {
            }
          }
        }
      }
      n94 = Build Array(w220, w219) -> (w218:cluster{"Resource Output":i32, "Position":i32}[])
    }
    frame #5 {
      n95 = Unbundle By Name(w239) -> ("Motion System"=w240:T7)
      n96 = case shown="\"NI 735x\", Default" w240 {
        tunnel: w239 -> [w241 w251 _]
        frame "NI 735x", Default {
          n97 = Unbundle By Name(w241) -> ("Motion Bd ID"=w243:u8, "# Axis"=w242:i8)
          n98 = call "CheckLimStat.vi"("# Axis"=w242, "Motion Board ID"=w243) -> ()  [unwired: 4 in]
        }
        frame "Galil" {
          n99 = Unbundle By Name(w251) -> ("GL Ref Out"=w248:refnum<k7>, "# Axis"=w249:i8)
          n100 = call "GL Command Set.vi"("Command"=Command_Menu."Status", "Axis"=w249, "Galil.IGalil"=w248) -> ("Response#"=w245:i32)  [unwired: 4 in, 4 out]
          n101 = In Range and Coerce(upper limit=3, x=w245, lower limit=2) -> (In Range?=w244:bool)  [unwired: 1 out]
          n102 = case shown="True" w244 {
            frame False {
            }
            frame True {
              n103 = One Button Dialog(message="A limit switch has been hit. Abort scan and reposition") -> ()  [unwired: 1 in, 1 out]
            }
          }
        }
        frame "Newport ESP", "No Motion Card" {
        }
      }
    }
    frame #6 {
      # "Set up trigs for pulse inversion trigger. Pegged to digitizer delays"
      n104 = case shown="1" w257 {
        tunnel: w254 -> [_ _ w260]
        frame 0 {
        }
        frame 1 {
          # "Set up trigs for prospective mode using counter 1. Now using PFI11 for gate of trigger and there is a seperate input line for EKG or equivalent sources"
          n105 = call "ProspectivePulseTrain.vi"() -> ()  [unwired: 2 in, 4 out]
        }
        frame 2, Default {
          (unwired) 4 items=["verify"=2, "reserve"=4, "commit"=3, "unreserve"=5, "abort"=6] ("action")
          w261 = 10123 items=["Finite Samples"=10178, "Continuous Samples"=10123] ("sample mode")
          # "Sets up CTR1 to generate pulse train on software trigger. Use for IQ trigger mode."
          n106 = Multiply(x=w260, y=1000) -> (x*y=w263:dbl)
          n107 = call-poly <vilib>:"DAQmx Create Virtual Channel.vi"("frequency"=w263, "duty cycle"=0.2, "counter"=tag "Dev1/ctr1") -> ("task out"=w265:refnum<k21>, "error out"=w266:errorcluster)  [unwired: 11 in]
          n108 = call-poly <vilib>:"DAQmx Timing.vi"("task/channels in"=w265, "sample mode"=w261, "error in"=w266) -> ("task out"=w258:refnum<k21>)  [unwired: 11 in, 1 out]
          n109 = global write "MotionGlobals.vi" "DAQmx Task 1"(w258) -> ()
        }
      }
      n110 = case shown="True" w255 {
        tunnel: w253 -> [_ w267]
        frame False {
        }
        frame True {
          (unwired) 5 ("Output Pulse#")
          # "CTR1 gate is feed from NI trig in"
          # "Use counter 0 gate if dividing EKG trigger"
          n111 = global read "MotionGlobals.vi" "Multi Trig#"() -> (w269:i32)
          n112 = call "MultiTrigBurst.vi"("high time"=0.00022, "Digitizer Settings"=w267, "Output Pulse#"=w269) -> ()  [unwired: 3 in, 2 out]
        }
      }
      n113 = Tick Count (ms)() -> (millisecond timer value=w256:u32)
    }
    frame #7 {
      # "Set up timing card for single pass pulser. Need four more triggers. Standard trigger for card one and then remaingin 4 channels  each have a trigger.  CT0, 2,3,4,5 send out pulses to trigger the pulser channels and they all pass through an OR GATE to trigger digitizers. Also take care of M mode and 1T - 5R modes."
      n114 = Unbundle By Name(w273) -> ("Dig Config"=w272:T12)
      n115 = case shown="\"5-CH pulser w/ ann array\"" w272 {
        tunnel: w276 -> [_ w287 _]
        tunnel: w275 -> [_ w288 w324]
        tunnel: [_ w285 _] -> w274
        tunnel: w273 -> [_ w282 w326]
        tunnel: w271 -> [_ w277 w323]
        tunnel: w270 -> [_ w280 w327]
        frame "Single channel", Default {
        }
        frame "5-CH pulser w/ ann array" {
          # "Prime Counters.\nHave to use alternate method\nwhen not using NI motion card."
          # "Start Counters"
          # "May need to spread out pulse with extra time for testing with a single pulser"
          n116 = Unbundle By Name(w280) -> ("Xmt/Rcv.XMIT"=w279:bool[])
          n117 = Not(x=w287) -> (.not. x?=w278:bool)
          n118 = call "5ChPulserTrigsNew.vi"("Motion Settings"=w277, "Digitizer Settings"=w282, "XMIT"=w279, "Axis"=w288, "M-mode?"=w278) -> ("5CH Pulser Tasks"=w285:refnum<k21>[])  [unwired: 4 in, 1 out]
          n119 = for {
            tunnel: w285 -> [w322] mode=indexing
            tunnel: [w321] -> w284
            n120 = call <vilib>:"DAQmx Start Task.vi"("task/channels in"=w322) -> ("error out"=w321:errorcluster)  [unwired: 1 in, 13 out]
          }
          n121 = for {
            tunnel: bool[][] [[TRUE], [FALSE]] ("data") -> [w313] mode=indexing
            tunnel: w284 -> [w311]
            tunnel: [w310] -> w283
            n122 = flat-sequence {
              tunnel: w313 -> [w317]
              tunnel: [w317] -> w314
              tunnel: [w315] -> w312
              tunnel: w311 -> [w315]
              tunnel: w314 -> [w320]
              tunnel: w312 -> [w319]
              tunnel: [w318] -> w310
              frame #0 {
                n123 = Wait (ms)(milliseconds to wait=u32 50) -> ()  [unwired: 1 out]
              }
              frame #1 {
                n124 = call "DAQ Assistant2"("data"=w320, "error in"=w319) -> ("error out"=w318:errorcluster)  [unwired: 16 in, 1 out]
              }
            }
          }
          n125 = Unbundle By Name(w277) -> ("Motion System"=w281:T7)
          n126 = case shown="\"Galil\"" w281 {
            tunnel: w283 -> [w291 w298 w302]
            tunnel: w277 -> [w290 w297 _]
            frame "NI 735x", Default {
              n127 = Unbundle By Name(w290) -> ("Motion Bd ID"=w289:u8)
              n128 = for {
                N: 3 -> [_]
                tunnel: w289 -> [w295]
                tunnel: [w294] -> _
                tunnel: w291 -> [w293]
                n129 = call "ForceBreakPt.vi"("error in"=w293, "Bd ID in"=w295) -> ("error out"=w294:errorcluster)  [unwired: 1 out]
              }
            }
            frame "Galil" {
              n130 = Unbundle By Name(w297) -> ("GL Ref Out"=w296:refnum<k7>)
              n131 = for {
                N: 3 -> [_]
                tunnel: w296 -> [w301]
                tunnel: w298 -> [w300]
                n132 = call "GL_ForceBreakPt.vi"("error in"=w300, "GL Ref Out"=w301) -> ()  [unwired: 2 out]
              }
            }
            frame "No Motion Card" {
              n133 = stacked-sequence {
                tunnel: refnum<k21> "QuantFlipFlop" ("task/channels in") -> [w306 _ w309]
                tunnel: w302 -> [w304 _ _]
                frame #0 {
                  n134 = call-poly <vilib>:"DAQmx Write.vi"("task/channels in"=w306, "data"=TRUE, "error in"=w304) -> ()  [unwired: 10 in, 3 out]
                }
                frame #1 {
                  n135 = Wait (ms)(milliseconds to wait=u32 500) -> ()  [unwired: 1 out]
                }
                frame #2 {
                  n136 = call-poly <vilib>:"DAQmx Write.vi"("task/channels in"=w309, "data"=FALSE) -> ()  [unwired: 11 in, 3 out]
                }
              }
            }
          }
        }
        frame "5-CH Pulser New" {
          # "2021 Version of daxsonics has built in triggering"
          n137 = Unbundle By Name(w327) -> ("Xmt/Rcv.XMIT"=w325:bool[])
          n138 = call "DaxInternaMultiTrig.vi"("Motion Settings"=w323, "Digitizer Settings"=w326, "XMIT"=w325, "Axis"=w324) -> ()  [unwired: 6 in, 1 out]
        }
      }
    }
    frame #8 {
      # "Remove AI feature. Never used"
      n139 = global read "MotionGlobals.vi" "DAQ Range"() -> (w330:cluster{"Max V":dbl, "Min V":dbl})
      n140 = Unbundle(w330) -> ("Max V"=w329:dbl, "Min V"=w328:dbl)
      n141 = case shown="13" w332 {
        tunnel: w334 -> [_ w343 w353]
        tunnel: w333 -> [_ w342 w365]
        tunnel: [_ w337 w362] -> w331
        tunnel: w329 -> [_ w336 w361]
        tunnel: w328 -> [_ w335 w360]
        frame 0, Default {
        }
        frame 13 {
          w340 = 3 items=["verify"=2, "reserve"=4, "commit"=3, "unreserve"=5, "abort"=6] ("action")
          w341 = 10083 items=["default"=-1, "RSE"=10083, "NRSE"=10078, "Differential"=10106, "Pseudodifferential"=12529] ("input terminal configuration")
          w347 = 10178 items=["Finite Samples"=10178, "Continuous Samples"=10123, "Hardware Timed Single Point"=12522] ("sample mode")
          # "Prep DAQ card to acquire on AI0"
          n142 = expression code="x*1000"(w342) -> (w346:dbl)
          n143 = call-poly <vilib>:"DAQmx Create Virtual Channel.vi"("maximum value"=w336, "minimum value"=w335, "input terminal configuration"=w341, "physical channels"=tag "Dev1/ai0") -> ("task out"=w344:refnum<k21>, "error out"=w349:errorcluster)  [unwired: 5 in, 5 out]
          n144 = call-poly <vilib>:"DAQmx Timing.vi"("task/channels in"=w344, "sample mode"=w347, "samples per channel"=w343, "rate"=w346, "source"=tag "/Dev1/PFI13", "error in"=w349) -> ("task out"=w339:refnum<k21>, "error out"=w338:errorcluster)  [unwired: 1 in, 7 out]
          n145 = call <vilib>:"DAQmx Control Task.vi"("task/channels in"=w339, "action"=w340, "error in"=w338) -> ("task out"=w337:refnum<k21>)  [unwired: 12 out]
        }
        frame 14 {
          w352 = 24000.0
          w363 = 3 items=["verify"=2, "reserve"=4, "commit"=3, "unreserve"=5, "abort"=6] ("action")
          w364 = 10083 items=["default"=-1, "RSE"=10083, "NRSE"=10078, "Differential"=10106, "Pseudodifferential"=12529] ("input terminal configuration")
          w368 = 10178 items=["Finite Samples"=10178, "Continuous Samples"=10123, "Hardware Timed Single Point"=12522] ("sample mode")
          # "Prep DAQ card to acquire on AI0 and AI1"
          n146 = expression code="1/(x*1000)"(w365) -> (w350:dbl)
          n147 = call-poly <vilib>:"DAQmx Create Virtual Channel.vi"("maximum value"=w361, "minimum value"=w360, "input terminal configuration"=w364, "physical channels"=tag "Dev1/ai0:1") -> ("task out"=w366:refnum<k21>, "error out"=w369:errorcluster)  [unwired: 5 in, 5 out]
          n148 = Compound Arithmetic op=MULTIPLY(w353, w350, w352) -> (w351:dbl)
          n149 = call-poly <vilib>:"DAQmx Timing.vi"("task/channels in"=w366, "sample mode"=w368, "samples per channel"=w351, "rate"=w352, "source"=tag "OnboardClock", "error in"=w369) -> ("task out"=w355:refnum<k21>, "error out"=w356:errorcluster)  [unwired: 1 in, 7 out]
          n150 = call-poly <vilib>:"DAQmx Trigger.vi"("task/channels in"=w355, "source"=tag "/Dev1/PFI13", "error in"=w356) -> ("task out"=w358:refnum<k21>, "error out"=w357:errorcluster)  [unwired: 1 in, 10 out]
          n151 = call <vilib>:"DAQmx Control Task.vi"("task/channels in"=w358, "action"=w363, "error in"=w357) -> ("task out"=w362:refnum<k21>)  [unwired: 12 out]
        }
      }
    }
    frame #9 {
      n152 = Unbundle By Name(w371) -> ("Full Array Scan?"=w370:bool)
      n153 = global read "SwitchGlobals.vi" "Switch Unit"() -> (w372:T23)
      n154 = case shown="False" w370 {
        tunnel: w372 -> [_ w373]
        frame False {
        }
        frame True {
          n155 = case shown="\"Pickering\", Default" w373 {
            frame "Cytex" {
              n156 = call "Cytex.vi"("Xmit Ring"=i8 1) -> ()  [unwired: 2 in, 3 out]
            }
            frame "Pickering", Default {
            }
          }
        }
      }
    }
    frame #10 {
      # "Temp array to store data to save memory. Only used in Synth Focus mode."
      # "Set up reference to data array. Used for \nsynth focusing"
      n157 = Unbundle By Name(w376) -> ("Synth Foc?"=w377:bool)
      n158 = case shown="False" w377 {
        tunnel: [w393 w405] -> w380
        tunnel: w382 -> [_ w397]
        tunnel: w381 -> [w392 w404]
        tunnel: w376 -> [w390 w400]
        tunnel: [w384 w399] -> w375
        frame False {
          n159 = Unbundle By Name(w390) -> ("downfactor"=w388:i32)
          n160 = Unbundle By Name(w392) -> ("lines per plane"=w389:i32, "rf points per line"=w387:i32)
          n161 = Divide(x=w387, y=w388) -> (x/y=w386:dbl)
          n162 = Initialize Array(i16 0, w389, w387) -> (w395:i16[][])
          n163 = Initialize Array(i16 0, w389, w386) -> (w385:i16[][])
          n164 = New Data Value Reference(data value=w395) -> (data value reference=w393:refnum<data-value>)  [unwired: 1 in, 1 out]
          n165 = New Data Value Reference(data value=w385) -> (data value reference=w384:refnum<data-value>)  [unwired: 1 in, 1 out]
        }
        frame True {
          n166 = Unbundle By Name(w404) -> ("rf points per line"=w398:i32)
          n167 = Unbundle By Name(w400) -> ("downfactor"=w403:i32)
          n168 = Divide(x=w398, y=w403) -> (x/y=w402:dbl)
          n169 = Initialize Array(i16 0, w397, w402) -> (w401:i16[][])
          n170 = Initialize Array(i16 0, w397, w398) -> (w406:i16[][])
          n171 = New Data Value Reference(data value=w401) -> (data value reference=w399:refnum<data-value>)  [unwired: 1 in, 1 out]
          n172 = New Data Value Reference(data value=w406) -> (data value reference=w405:refnum<data-value>)  [unwired: 1 in, 1 out]
        }
      }
      n173 = case shown="True" w378 {
        frame False {
        }
        frame True {
          # "Open feedback display if 2D"
          n174 = case shown="True" FALSE {
            frame False {
            }
            frame True {
              n175 = call "ClosePopUpWindow.vi"() -> ()  [unwired: 12 in]
            }
          }
        }
      }
      n176 = Bundle By Name(cluster=w381, "Data Ref RF"=w380, "Data Ref Log"=w375) -> (w379:T10)
    }
    frame #11 {
      n177 = call "GetAxisCount.vi"("Motion Settings"=w413, "Scan Axis"=w416) -> ("Counts"=w415:dbl)  [unwired: 9 in]
      n178 = for {
        N: w420 -> [_]
        tunnel: w433 -> [w459]
        tunnel: w432 -> [w458]
        tunnel: w431 -> [w457]
        tunnel: [w456] -> w430 mode=indexing
        tunnel: w429 -> [w455]
        tunnel: w428 -> [w454]
        tunnel: w416 -> [w453]
        tunnel: [w452] -> w427 mode=indexing
        tunnel: w426 -> [w451]
        tunnel: w425 -> [w450]
        tunnel: w424 -> [w449]
        tunnel: w423 -> [w448]
        tunnel: w422 -> [w447]
        tunnel: w415 -> [w446]
        tunnel: [w445] -> w421
        tunnel: w419 -> [w444]
        tunnel: w418 -> [w442]
        tunnel: w417 -> [w441]
        tunnel: w412 -> [w440]
        tunnel: w414 -> [w439]
        tunnel: w413 -> [w438]
        tunnel: w411 -> [w437]
        tunnel: w410 -> [w436]
        tunnel: w409 -> [w435]
        tunnel: w408 -> [w434]
        i -> [w443]
        n179 = stacked-sequence {
          seq-local: [w464 _ _] -> [_ w482 _]
          seq-local: [_ w481 _] -> [_ _ w756]
          tunnel: w459 -> [_ w497 _]
          tunnel: w458 -> [_ w496 _]
          tunnel: w457 -> [_ w495 _]
          tunnel: [_ w494 _] -> w456
          tunnel: w455 -> [_ w493 _]
          tunnel: w454 -> [_ w492 w761]
          tunnel: w453 -> [_ w491 w764]
          tunnel: [_ w490 _] -> w452
          tunnel: w451 -> [_ w489 _]
          tunnel: w450 -> [_ w488 _]
          tunnel: w449 -> [_ w487 _]
          tunnel: w448 -> [_ w486 w762]
          tunnel: w447 -> [w463 _ _]
          tunnel: w446 -> [_ w485 _]
          tunnel: [_ w484 _] -> w445
          tunnel: w444 -> [_ _ w763]
          tunnel: w443 -> [w462 w477 _]
          tunnel: w442 -> [_ _ w760]
          tunnel: w441 -> [_ _ w759]
          tunnel: w439 -> [_ _ w758]
          tunnel: w440 -> [_ w480 _]
          tunnel: w438 -> [w461 w479 w754]
          tunnel: w437 -> [_ w478 _]
          tunnel: w436 -> [_ w476 _]
          tunnel: w435 -> [_ w475 _]
          tunnel: w434 -> [_ w474 _]
          frame #0 {
            n180 = Unbundle By Name(w461) -> ("Add Axis"=w460:bool)
            n181 = case shown="True" w460 {
              tunnel: [w465 w468] -> w464
              tunnel: w463 -> [w465 w466]
              tunnel: w462 -> [_ w467]
              frame False {
              }
              frame True {
                w472 = ""
                # "Modify file name for 3D retro acquisition. Insert 3DR and number just before last a"
                n182 = call "NumberFileName.vi"("String"=w472, "Digits"=3, "File number"=w467, "file name"=w472) -> ("Numbered File"=w470:string)
                n183 = Concatenate Strings(w466, "x3D" ("string"), w470, "a" ("string")) -> (w468:string)
              }
            }
          }
          frame #1 {
            n184 = for {
              N: w488 -> [_]
              tunnel: w495 -> [w525]
              tunnel: w497 -> [w524]
              tunnel: w492 -> [w523]
              tunnel: w496 -> [w522]
              tunnel: w491 -> [w521]
              shift-right: [w516] -> _
              shift-left: FALSE ("reverse") -> [w514]
              tunnel: w493 -> [w520]
              tunnel: [w519] -> w494 mode=indexing
              tunnel: w489 -> [w518]
              tunnel: [w517] -> w490 mode=indexing
              tunnel: w487 -> [w515]
              tunnel: w486 -> [w506]
              tunnel: w485 -> [w512]
              tunnel: [w511] -> w484
              tunnel: w482 -> [w510]
              tunnel: [w509] -> w481
              tunnel: w480 -> [w502]
              tunnel: w479 -> [w508]
              tunnel: w478 -> [w505]
              tunnel: w477 -> [w504]
              tunnel: w476 -> [w503]
              tunnel: w475 -> [w499]
              tunnel: w474 -> [w498]
              i -> [w507]
              n185 = Bundle By Name(cluster=w508, "Plane"=w507) -> (w501:T6)
              n186 = call "StopScan.vi"("Motion Settings In"=w501, "Digitizer Settings"=w502) -> ("Stop Now? Dup"=w500:bool)  [unwired: 4 in]
              n187 = Decrement(x=w506) -> (x-1=w513:i32)
              n188 = stacked-sequence {
                seq-local: [_ _ w601 _ _ _ _] -> [_ _ _ _ w685 _ _]
                seq-local: [w535 _ _ _ _ _ _] -> [_ w578 w595 w643 _ _ _]
                tunnel: w525 -> [_ _ w611 _ _ _ _]
                tunnel: w524 -> [_ _ w612 _ _ _ _]
                tunnel: w523 -> [w529 _ _ _ w689 _ _]
                tunnel: w522 -> [_ _ w614 _ w688 _ _]
                tunnel: w521 -> [_ _ w600 _ _ _ _]
                tunnel: w514 -> [_ _ w608 _ _ _ _]
                tunnel: w520 -> [_ _ w615 _ _ _ _]
                tunnel: [_ _ w609 _ _ _ _] -> w519
                tunnel: w518 -> [_ _ w613 w645 _ _ _]
                tunnel: [_ _ w610 _ _ _ _] -> w517
                tunnel: [_ _ w602 _ _ _ _] -> w511
                tunnel: [_ _ w603 _ _ _ _] -> w516
                tunnel: w515 -> [_ _ w607 _ _ _ _]
                tunnel: w507 -> [w536 w579 _ w648 w681 _ _]
                tunnel: w513 -> [w537 _ _ _ w686 _ _]
                tunnel: w510 -> [_ _ w605 w649 _ _ _]
                tunnel: w512 -> [_ _ w599 _ _ _ _]
                tunnel: [_ _ w601 _ _ _ _] -> w509
                tunnel: w502 -> [w533 _ _ _ _ w741 _]
                tunnel: w505 -> [_ _ w597 w646 _ _ _]
                tunnel: w504 -> [w532 _ _ _ _ _ _]
                tunnel: w503 -> [w530 _ _ _ _ _ _]
                tunnel: w501 -> [w528 _ w594 w644 w684 _ w748]
                tunnel: w500 -> [_ w577 _ _ w683 _ _]
                tunnel: w499 -> [_ _ _ _ w682 _ _]
                tunnel: w498 -> [_ _ w593 _ _ _ _]
                frame #0 {
                  n189 = Unbundle By Name(w533) -> ("Fix Z Delay?"=w534:bool)
                  n190 = And(x=w534, y=w530) -> (x .and. y?=w531:bool)
                  n191 = case shown="True" w531 {
                    tunnel: w537 -> [_ w561]
                    tunnel: w536 -> [_ w563]
                    tunnel: [w538 w570] -> w535
                    tunnel: w533 -> [w538 w569]
                    tunnel: w528 -> [_ w568]
                    tunnel: w532 -> [_ w562]
                    tunnel: w529 -> [_ w545]
                    frame False {
                    }
                    frame True {
                      # "Shift delay to maintain window depth. Need twice the linear distance to find delay. This is only meant for use with a set of Z planes"
                      n192 = Unbundle By Name(w568) -> ("Xtra planes"=w559:i32, "Xtra plane\ndistance  (um)"=w567:i32, "Add Axis"=w557:bool, "Distance between\nscan planes (um)"=w565:sgl, "Reverse Z axis?"=w547:bool)
                      n193 = Unbundle By Name(w569) -> ("Digitizer delay (us)"=w542:dbl, "One Way Transmission?"=w552:bool)
                      n194 = global read "MotionGlobals.vi" "c mm/mics"() -> (w548:sgl)
                      n195 = Select(t=1.0, s=w552, f=0.5) -> (s? t:f=w549:dbl)
                      n196 = Decrement(x=w559) -> (x-1=w558:i32)
                      n197 = Select(t=w562, s=w557, f=w563) -> (s? t:f=w564:i32)
                      n198 = Multiply(x=w549, y=w548) -> (x*y=w571:dbl)
                      n199 = Select(t=w567, s=w557, f=w565) -> (s? t:f=w566:sgl)
                      n200 = Select(t=w558, s=w557, f=w561) -> (s? t:f=w560:i32)
                      n201 = Reciprocal(x=w571) -> (1/x=w572:dbl)
                      n202 = Divide(x=w560, y=-2) -> (x/y=w574:dbl)
                      n203 = Add(x=w574, y=w564) -> (x+y=w573:dbl)
                      n204 = Equal?(x=w545, y=3) -> (x = y?=w544:bool)
                      n205 = Multiply(x=w573, y=w566) -> (x*y=w556:dbl)
                      n206 = And(x=w547, y=w544) -> (x .and. y?=w546:bool)
                      n207 = Negate(x=w556) -> (-x=w553:dbl)
                      n208 = Negate(x=w553) -> (-x=w554:dbl)
                      n209 = Select(t=w553, s=w546, f=w554) -> (s? t:f=w555:dbl)
                      n210 = Compound Arithmetic op=MULTIPLY(w572, w555, 0.001) -> (w540:dbl)
                      n211 = global write "MotionGlobals.vi" "Preview Configed?"(FALSE ("Popped Up Before?")) -> ()
                      n212 = Compound Arithmetic op=ADD(w542, w540) -> (w541:dbl)
                      n213 = Bundle By Name(cluster=w569, "Digitizer delay (us)"=w541) -> (w570:T10)
                    }
                  }
                }
                frame #1 {
                  n214 = case shown="False" w577 {
                    tunnel: w579 -> [w584 _]
                    tunnel: w578 -> [w580 _]
                    frame False {
                      n215 = global read "MotionGlobals.vi" "Breath Trig"() -> (w582:T24)
                      n216 = Quotient & Remainder(x=w584, y="Breath Divide") -> (x-y*floor(x/y)=w583:i32)  [unwired: 1 out]
                      n217 = case shown="0" w583 {
                        tunnel: w582 -> [w586 _]
                        tunnel: w580 -> [w585 _]
                        frame 0 {
                          # "Use Ring 1 to track respiratory motion"
                          n218 = case shown="1, Default" w586 {
                            tunnel: [_ w589 w592] -> _
                            tunnel: 0 -> [_ _ w591]
                            tunnel: w585 -> [_ _ w590]
                            frame 0 {
                            }
                            frame 3 {
                              n219 = global read "MotionGlobals.vi" "Resp Wait (ms)"() -> (w588:u32)
                              n220 = call "BIOPAC breath gating.vi"("Resp Wait (ms)"=w588) -> ("Resp Gate"=w589:bool)  [unwired: 2 in]
                            }
                            frame 1, Default {
                              # "Trigger after breath motion artifact."
                              n221 = call "BreathTrig.vi"("Digitizer Settings"=w590, "Xmit Ring"=w591) -> ("BINGO"=w592:bool)  [unwired: 4 in, 5 out]
                            }
                          }
                        }
                        frame 1, Default {
                        }
                      }
                    }
                    frame True {
                    }
                  }
                }
                frame #2 {
                  # "All Data Acq now takes plce here"
                  n222 = Unbundle By Name(w597) -> ("Full Array Scan?"=w596:bool)
                  n223 = Unbundle By Name(w595) -> ("Total Dig CH"=w598:i32)
                  n224 = Select(t=w598, s=w596, f=1) -> (s? t:f=w606:i32)
                  n225 = for {
                    N: w606 -> [_]
                    shift-right: [w642] -> w603
                    shift-left: w608 -> [w641]
                    tunnel: w615 -> [w628]
                    tunnel: w600 -> [w640]
                    tunnel: w614 -> [w639]
                    tunnel: w613 -> [w638]
                    tunnel: w612 -> [w637]
                    tunnel: w611 -> [w636]
                    tunnel: [w635] -> w610
                    tunnel: [w634] -> w609
                    tunnel: w596 -> [w627]
                    tunnel: w607 -> [w631]
                    tunnel: w599 -> [w629]
                    tunnel: w605 -> [w630]
                    shift-right: [w621] -> _
                    shift-left: i32[] [0] -> [w626]
                    tunnel: [w624] -> w602
                    tunnel: [w623] -> w601
                    shift-right: [w620] -> _
                    shift-left: w595 -> [w622]
                    tunnel: w597 -> [w619]
                    tunnel: w594 -> [w618]
                    tunnel: w593 -> [w617]
                    i -> [w633]
                    n226 = Select(t=w633, s=w627, f=w631) -> (s? t:f=w632:i32)
                    n227 = call "DataAcqMaster.vi"("Motion Settings In"=w618, "2-D motor"=w639, "Type of scan"=w638, "Move motor"=w637, "Therapy (T)"=w636, "Scan Name"=w630, "Xmit Ring"=w632, "Digitizer Settings"=w622, "lines per plane mod"=w628, "Ann Array Params"=w619, "Reverse ?"=w641, "DAQmx Task 2"=w617, "Full Array Scan?"=w627, "start value"=w629, "scan axis"=w640) -> ("Stop Scan"=w623:bool, "Motion error"=w635:bool, "Timeout"=w634:bool, "error out"=w624:errorcluster, "Record Index"=w625:i32)  [unwired: 3 in, 5 out]
                    n228 = Not(x=w641) -> (.not. x?=w642:bool)
                    n229 = Build Array (concatenate)(w626, w625) -> (w621:i32[])
                    n230 = Bundle By Name(cluster=w622, "Bulk Start Indexes"=w621) -> (w620:T10)
                  }
                }
                frame #3 {
                  # "Save synthetic focused data to temp file"
                  n231 = Unbundle By Name(w646) -> ("Synth Foc?"=w647:bool)
                  n232 = case shown="True" w647 {
                    tunnel: w649 -> [_ w652]
                    tunnel: w648 -> [_ w651]
                    tunnel: w643 -> [_ w661]
                    tunnel: w644 -> [_ w656]
                    tunnel: w646 -> [_ w655]
                    tunnel: w645 -> [_ w653]
                    frame False {
                    }
                    frame True {
                      n233 = Unbundle By Name(w661) -> ("Data Ref RF"=w660:refnum<data-value>, "Voltage Scale"=w659:dbl, "bits A/D"=w658:i8, "Data Ref Log"=w654:refnum<data-value>)
                      n234 = call "VScaleInfoNI.vi"("A/D bits"=w658, "gain"=w659) -> ("Voltage Scale"=w657:T25)  [unwired: 5 in, 3 out]
                      n235 = Unbundle By Name(w655) -> ("Save TIFF?"=w650:bool)
                      n236 = in-place {
                        in-place-border: w651 -> [w676]
                        in-place-border: w652 -> [w680]
                        in-place-border: w661 -> [w674]
                        in-place-border: w656 -> [w675]
                        in-place-border: w657 -> [w679]
                        in-place-border: w655 -> [w672]
                        in-place-border: w653 -> [w671]
                        n237 = in-place-dvr #1(w660) -> (w677:i16[][])  [unwired: 1 out]
                        n238 = expression code="x*0"(w677) -> (w678:i16[][])
                        n239 = call "SaveSFData.vi"("File Name"=w680, "Current Plane"=w676, "Digitizer Settings"=w674, "Motion Settings"=w675, "Voltage scaling"=w679, "Ann Array Params"=w672, "Data In"=w677, "Type of scan"=w671) -> ()  [unwired: 1 in]
                        n240 = call "PopUpDisplay.vi"("Data"=w677, "Plane"=w676, "Motion Settings In"=w675, "Digitizer Settings"=w674, "virtual T/R Pairs"=25) -> ()  [unwired: 11 in]
                        n241 = in-place-dvr #1(w678) -> ()  [unwired: 2 out]
                      }
                      n242 = case shown="True" w650 {
                        tunnel: w654 -> [_ w665]
                        tunnel: w652 -> [_ w662]
                        tunnel: w651 -> [_ w664]
                        tunnel: w653 -> [_ w663]
                        frame False {
                        }
                        frame True {
                          n243 = in-place {
                            in-place-border: w664 -> [w667]
                            in-place-border: w663 -> [w666]
                            in-place-border: w662 -> [w669]
                            n244 = in-place-dvr #2(w665) -> (w668:i16[][])  [unwired: 1 out]
                            n245 = call "SaveTIFF.vi"("Type of scan"=w666, "File Name"=w669, "Data In"=w668, "Current Plane"=w667) -> ()  [unwired: 8 in]
                            n246 = expression code="x*0"(w668) -> (w670:i16[][])
                            n247 = in-place-dvr #2(w670) -> ()  [unwired: 2 out]
                          }
                        }
                      }
                    }
                  }
                }
                frame #4 {
                  # "Move to new scan plane in necessary"
                  n248 = Equal?(x=w686, y=w681) -> (x = y?=w687:bool)
                  n249 = case shown="True" w688 {
                    tunnel: w689 -> [_ w697]
                    tunnel: w687 -> [_ w696]
                    tunnel: w685 -> [_ w695]
                    tunnel: w684 -> [_ w694]
                    tunnel: w683 -> [_ w691]
                    tunnel: w682 -> [_ w693]
                    tunnel: w681 -> [_ w692]
                    frame False {
                    }
                    frame True {
                      n250 = Compound Arithmetic op=OR(w691, w696, w695) -> (w690:bool)
                      n251 = case shown="False" w690 {
                        tunnel: w697 -> [w701 _]
                        tunnel: w694 -> [w703 _]
                        tunnel: w693 -> [w699 _]
                        tunnel: w692 -> [w698 _]
                        frame False {
                          # "Skip if last scan"
                          n252 = Unbundle By Name(w703) -> ("Motion System"=w704:T7)
                          n253 = call "Find_Count_Step_Interval.vi"("BP Int (F)/Plane Int (T)"=TRUE, "Motion Settings In"=w703, "Axis"=w701) -> ("BP Interval"=w702:dbl)  [unwired: 7 in, 1 out]
                          n254 = case shown="\"Galil\"" w704 {
                            tunnel: w702 -> [_ w705 w714 w727 _]
                            tunnel: w701 -> [_ w710 w723 w729 _]
                            tunnel: [_ w709 _ _ _] -> _
                            tunnel: w703 -> [_ w708 w726 w728 _]
                            tunnel: w699 -> [_ _ w713 _ _]
                            tunnel: w698 -> [_ _ w715 _ _]
                            frame "MM3000" {
                            }
                            frame "NI 735x", Default {
                              n255 = Unbundle By Name(w708) -> ("Motion Bd ID"=w707:u8)
                              n256 = call "MoveMotor.vi"("Position Mode (Absolute)"=T18."Relative Position", "Target Position (0)"=w705, "Axis or Vector Space"=w710, "Motion Bd ID"=w707) -> ("error out"=w709:errorcluster)  [unwired: 5 in, 2 out]
                            }
                            frame "Galil" {
                              n257 = Unbundle By Name(w726) -> ("GL Ref Out"=w722:refnum<k7>)
                              n258 = Increment(x=w715) -> (x+1=w716:i32)
                              n259 = Multiply(x=w714, y=w716) -> (x*y=w712:dbl)
                              n260 = Decrement(x=w723) -> (x-1=w724:i32)
                              n261 = Add(x=w712, y=w713) -> (x+y=w711:dbl)
                              n262 = call "GL Set Operation Mode.vi"("position cts (abs/rel)"=w711, "Position Mode (Absolute)"=T18."Absolute Position", "Start Now?"=TRUE, "Axis"=w724, "Galil.IGalil"=w722) -> ("error out"=w719:errorcluster, "Axis Out Output"=w718:T19, "Galil Out"=w720:refnum<k7>)  [unwired: 4 in]
                              n263 = call "GL Position.vi"("Wait for Motion Complete"=TRUE, "error in (no error)"=w719, "Axis"=w718, "Galil.IGalil"=w720) -> ()  [unwired: 2 in, 4 out]
                            }
                            frame "Newport ESP" {
                              n264 = case shown="1, Default" w727 {
                                selector: w727 -> [_ w733]
                                tunnel: w729 -> [_ w734]
                                tunnel: w728 -> [_ w731]
                                frame 0 {
                                }
                                frame 1, Default {
                                n265 = Unbundle By Name(w731) -> ("ESP VISA"=w730:refnum<visa-resource-name>)
                                n266 = flat-sequence {
                                tunnel: w734 -> [w737]
                                tunnel: w733 -> [w736]
                                tunnel: [w738] -> w732
                                tunnel: w730 -> [w735]
                                tunnel: [w740] -> _
                                tunnel: w732 -> [w739]
                                frame #0 {
                                n267 = call <instrlib>:"Move Relative.vi"("Position (0 units)"=w736, "Axis (1)"=w737, "VISA resource name"=w735) -> ("VISA resource name out"=w738:refnum<visa-resource-name>)  [unwired: 3 in, 1 out]
                                }
                                frame #1 {
                                n268 = call "WaitStopEPS.vi"("VISA resource name"=w739) -> ("Stopped"=w740:bool)  [unwired: 2 in, 2 out]
                                }
                                }
                                }
                              }
                            }
                            frame "No Motion Card" {
                            }
                          }
                        }
                        frame True {
                        }
                      }
                    }
                  }
                }
                frame #5 {
                  n269 = Unbundle By Name(w741) -> ("Main Digitizer"=w742:T11)
                  n270 = case shown="\"NI Digitizer\"" w742 {
                    tunnel: w741 -> [_ w744 w746]
                    frame "Acqiris Digitizer", Default {
                    }
                    frame "LeCroy" {
                      n271 = Unbundle By Name(w744) -> ("Digitizer ID Cluster.LeCroy VISA"=w743:refnum<visa-resource-name>)
                      n272 = call <instrlib>:"Abort.vi"("VISA resource name"=w743) -> ()  [unwired: 9 in, 2 out]
                    }
                    frame "NI Digitizer" {
                      n273 = Unbundle By Name(w746) -> ("Digitizer ID Cluster.NI Instr Handles"=w745:refnum<k15>[])
                      n274 = for {
                        tunnel: w745 -> [w747] mode=indexing
                        n275 = call <instrlib>:"niScope Abort.vi"("instrument handle"=w747) -> ()  [unwired: 1 in, 14 out]
                      }
                    }
                  }
                }
                frame #6 {
                  n276 = Unbundle By Name(w748) -> ("Motion System"=w749:T7)
                  n277 = case shown="\"Newport ESP\", \"No Motion Card\", Default" w749 {
                    tunnel: w748 -> [w752 _]
                    frame "NI 735x" {
                      n278 = Unbundle By Name(w752) -> ("Motion Bd ID"=w751:u8, "# Axis"=w750:i8)
                      n279 = call "CheckLimStat.vi"("# Axis"=w750, "Motion Board ID"=w751) -> ()  [unwired: 4 in]
                    }
                    frame "Newport ESP", "No Motion Card", Default {
                    }
                  }
                }
              }
              n280 = case shown="False" w500 {
                tunnel: w501 -> [w527 _]
                frame False {
                  n281 = call "FindLocation.vi"("Motion Settings"=w527, "Wait for Motion Complete"=TRUE) -> ()  [unwired: 1 in, 4 out]
                }
                frame True {
                }
              }
              "Current Plane" <- w507
            }
          }
          frame #2 {
            n282 = Unbundle By Name(w754) -> ("Add Axis"=w753:bool)
            n283 = Not(x=w756) -> (.not. x?=w755:bool)
            n284 = And(x=w753, y=w755) -> (x .and. y?=w757:bool)
            n285 = case shown="True" w757 {
              tunnel: w764 -> [_ w774]
              tunnel: w763 -> [_ w779]
              tunnel: w762 -> [_ w777]
              tunnel: w761 -> [_ w769]
              tunnel: w760 -> [_ w771]
              tunnel: w759 -> [_ w773]
              tunnel: w758 -> [_ w770]
              tunnel: w754 -> [_ w766]
              frame False {
              }
              frame True {
                # "Take 2D stages back to start corner"
                # "Increment to next additional axis plane"
                n286 = call "Find_Count_Step_Interval.vi"("BP Int (F)/Plane Int (T)"=TRUE, "Motion Settings In"=w766, "Axis"=w769) -> ("BP Interval"=w768:dbl)  [unwired: 7 in, 1 out]
                n287 = Decrement(x=w777) -> (x-1=w778:i32)
                n288 = Unbundle By Name(w766) -> ("Motion System"=w765:T7)
                n289 = Multiply(x=w778, y=w768) -> (x*y=w776:dbl)
                n290 = Select(t=w774, s=w771, f=w773) -> (s? t:f=w772:i32)
                n291 = Negate(x=w776) -> (-x=w775:dbl)
                n292 = case shown="\"Galil\"" w765 {
                  tunnel: w779 -> [_ w789 w806]
                  tunnel: w775 -> [_ w787 w814]
                  tunnel: w772 -> [_ w785 w807]
                  tunnel: w771 -> [_ w784 w813]
                  tunnel: w770 -> [_ w783 w812]
                  tunnel: w766 -> [_ w781 w811]
                  tunnel: w769 -> [_ w780 w810]
                  frame "MM3000", Default {
                  }
                  frame "NI 735x" {
                    w786 = 1
                    n293 = Unbundle By Name(w781) -> ("Motion Bd ID"=w782:u8)
                    n294 = call "MoveMotor.vi"("Position Mode (Absolute)"=w786, "Target Position (0)"=w789, "Axis or Vector Space"=w785, "Motion Bd ID"=w782) -> ("error out"=w790:errorcluster, "Bd ID Out"=w788:u8)  [unwired: 5 in, 1 out]
                    n295 = case shown="False" w784 {
                      tunnel: w790 -> [_ w801]
                      tunnel: w788 -> [w791 w800]
                      tunnel: w780 -> [_ w799]
                      tunnel: w787 -> [_ w798]
                      tunnel: w786 -> [_ w797]
                      tunnel: w783 -> [w792 _]
                      frame False {
                        n296 = for {
                          tunnel: w792 -> [w796] mode=indexing
                          tunnel: w791 -> [w794]
                          n297 = Unbundle(w796) -> ("Resource Output"=w795:i32, "Position"=w793:i32)
                          n298 = call "MoveMotor.vi"("Target Position (0)"=w793, "Axis or Vector Space"=w795, "Motion Bd ID"=w794) -> ()  [unwired: 6 in, 3 out]
                        }
                      }
                      frame True {
                        # "Only for 3D retro. Move back down the retro scan axis and increment to next plane. Then repeat acquisition"
                        n299 = call "MoveMotor.vi"("Position Mode (Absolute)"=w797, "error in (no error)"=w801, "Target Position (0)"=w798, "Axis or Vector Space"=w799, "Motion Bd ID"=w800) -> ()  [unwired: 4 in, 3 out]
                      }
                    }
                  }
                  frame "Galil" {
                    n300 = Decrement(x=w807) -> (x-1=w808:i32)
                    n301 = Unbundle By Name(w811) -> ("GL Ref Out"=w805:refnum<k7>)
                    n302 = call "GL Set Operation Mode.vi"("position cts (abs/rel)"=w806, "Position Mode (Absolute)"=T18."Relative Position", "Start Now?"=TRUE, "Axis"=w808, "Galil.IGalil"=w805) -> ("error out"=w802:errorcluster, "Galil Out"=w803:refnum<k7>)  [unwired: 4 in, 1 out]
                    n303 = case shown="True" w813 {
                      tunnel: w810 -> [_ w829]
                      tunnel: w814 -> [_ w832]
                      tunnel: w812 -> [w816 _]
                      tunnel: w803 -> [w815 w831]
                      tunnel: w802 -> [_ w830]
                      frame False {
                        n304 = for {
                          tunnel: w816 -> [w822] mode=indexing
                          tunnel: w815 -> [w818]
                          n305 = Unbundle(w822) -> ("Resource Output"=w819:i32, "Position"=w821:i32)
                          n306 = Decrement(x=w819) -> (x-1=w820:i32)
                          n307 = call "GL Set Operation Mode.vi"("position cts (abs/rel)"=w821, "Start Now?"=TRUE, "Axis"=w820, "Galil.IGalil"=w818) -> ()  [unwired: 5 in, 3 out]
                        }
                      }
                      frame True {
                        # "Only for 3D retro. Move back down the retro scan axis and increment to next plane. Then repeat acquisition"
                        n308 = Decrement(x=w829) -> (x-1=w828:i32)
                        n309 = call "GL Set Operation Mode.vi"("position cts (abs/rel)"=w832, "Position Mode (Absolute)"=T18."Relative Position", "error in (no error)"=w830, "Start Now?"=TRUE, "Axis"=w828, "Galil.IGalil"=w831) -> ("error out"=w824:errorcluster, "Axis Out Output"=w823:T19, "Galil Out"=w825:refnum<k7>)  [unwired: 3 in]
                        n310 = call "GL Position.vi"("error in (no error)"=w824, "Axis"=w823, "Galil.IGalil"=w825) -> ()  [unwired: 3 in, 4 out]
                      }
                    }
                  }
                }
              }
            }
          }
        }
      }
    }
    frame #12 {
      n311 = Unbundle By Name(w834) -> ("Motion System"=w835:T7)
      n312 = Unbundle By Name(w834) -> ("Motor Parameters.velocity ct/s"=w841:dbl[], "Motor Parameters.accel ct/s^2"=w840:dbl[])
      n313 = Decrement(x=w838) -> (x-1=w839:i32)
      n314 = Index Array(array=w841, index=w839) -> (element=w836:dbl)
      n315 = Index Array(array=w840, index=w839) -> (element=w837:dbl)
      n316 = case shown="\"Galil\"" w835 {
        tunnel: w838 -> [_ w842 w862 w886]
        tunnel: w837 -> [_ w845 w864 w884]
        tunnel: w836 -> [_ w844 w863 w883]
        tunnel: w834 -> [_ w843 w860 w882]
        frame "MM3000", "No Motion Card" {
        }
        frame "NI 735x", Default {
          n317 = disable-structure shown="Disabled" {
            disable-tunnel: w845 -> [w851 _]
            disable-tunnel: w844 -> [w850 _]
            disable-tunnel: w843 -> [w849 _]
            disable-tunnel: w842 -> [w848 _]
            frame Disabled {
              # "Return Velocity to pre-scan value (for cases with real slow frame rate) except for SMAC"
              n318 = Unbundle By Name(w849) -> ("SMAC Axis"=w847:u16, "Motion Bd ID"=w846:u8)
              n319 = Equal?(x=w848, y=w847) -> (x = y?=w852:bool)
              n320 = case shown="False" w852 {
                tunnel: w848 -> [w856 _]
                tunnel: w851 -> [w855 _]
                tunnel: w850 -> [w854 _]
                tunnel: w846 -> [w853 _]
                frame False {
                  n321 = call <vilib>:"Load Velocity.flx"("Velocity (10000)"=w854, "Axis or Vector Space"=w856, "Board ID"=w853) -> ("error out"=w858:errorcluster, "Resource Output"=w857:T22, "Bd ID Out"=w859:T26)  [unwired: 4 in]
                  n322 = call "Load Acceleration/Deceleration.flx"("Acceleration (100000)"=w855, "error in (no error)"=w858, "Axis or Vector Space"=w857, "Board ID"=w859) -> ()  [unwired: 3 in, 3 out]
                }
                frame True {
                }
              }
            }
            frame Enabled {
            }
          }
        }
        frame "Galil" {
          # "Return Velocity to pre-scan value (for cases with real slow frame rate) except for SMAC"
          n323 = Unbundle By Name(w860) -> ("SMAC Axis"=w861:u16)
          n324 = Equal?(x=w862, y=w861) -> (x = y?=w865:bool)
          n325 = case shown="False" w865 {
            tunnel: w862 -> [w879 _]
            tunnel: w864 -> [w871 _]
            tunnel: w863 -> [w877 _]
            tunnel: w860 -> [w880 _]
            frame False {
              n326 = Unbundle By Name(w880) -> ("GL Ref Out"=w878:refnum<k7>)
              n327 = Decrement(x=w879) -> (x-1=w872:i32)
              n328 = call "GL Command Set.vi"("Command"=Command_Menu."Velocity", "Value"=w877, "Axis"=w872, "Galil.IGalil"=w878) -> ("error out"=w875:errorcluster, "Axis Out"=w870:T19, "ref out"=w876:refnum<k7>)  [unwired: 3 in, 2 out]
              n329 = call "GL Command Set.vi"("Command"=Command_Menu."Acceleration", "error in (no error)"=w875, "Value"=w871, "Axis"=w870, "Galil.IGalil"=w876) -> ("error out"=w873:errorcluster, "Axis Out"=w869:T19, "ref out"=w874:refnum<k7>)  [unwired: 2 in, 2 out]
              n330 = call "GL Command Set.vi"("Command"=Command_Menu."Deceleration", "error in (no error)"=w873, "Value"=w871, "Axis"=w869, "Galil.IGalil"=w874) -> ()  [unwired: 2 in, 5 out]
            }
            frame True {
            }
          }
        }
        frame "Newport ESP" {
          n331 = Unbundle By Name(w882) -> ("ESP VISA"=w881:refnum<visa-resource-name>)
          n332 = call "WaitStopEPS.vi"("VISA resource name"=w881) -> ("VISA resource name out"=w885:refnum<visa-resource-name>)  [unwired: 2 in, 2 out]
          n333 = call <instrlib>:"Set Velocity.vi"("Velocity (units/s)"=w883, "Axis (1)"=w886, "VISA resource name"=w885) -> ("error out"=w887:errorcluster, "VISA resource name out"=w890:refnum<visa-resource-name>)  [unwired: 3 in]
          n334 = call <instrlib>:"Set Acceleration.vi"("error in (no error)"=w887, "Acceleration (0 units/s²)"=w884, "Axis (1)"=w886, "VISA resource name"=w890) -> ("error out"=w888:errorcluster, "VISA resource name out"=w889:refnum<visa-resource-name>)  [unwired: 2 in]
          n335 = call <instrlib>:"Set Deceleration.vi"("error in (no error)"=w888, "Deceleration (0 units/s²)"=w884, "Axis (1)"=w886, "VISA resource name"=w889) -> ()  [unwired: 2 in, 2 out]
        }
      }
      n336 = Tick Count (ms)() -> (millisecond timer value=w833:u32)
    }
    frame #13 {
      # "Return to start"
      # "Don't need to move z axis unless changes are made to program."
      n337 = Unbundle By Name(w892) -> ("# Axis"=w893:i8, "Motion System"=w894:T7)
      n338 = for {
        N: w893 -> [_]
        tunnel: [w899] -> w895 mode=indexing
        tunnel: w892 -> [w898]
        i -> [w897]
        n339 = Increment(x=w897) -> (x+1=w900:i32)
        n340 = call "GetAxisCount.vi"("Motion Settings"=w898, "Scan Axis"=w900) -> ("Counts"=w899:dbl)  [unwired: 9 in]
      }
      n341 = Array Subset(array=w895, length=w893) -> (w896:dbl[])  [unwired: 1 in]
      n342 = case shown="True" w891 {
        tunnel: w896 -> [_ w904]
        tunnel: w894 -> [_ w903]
        tunnel: w892 -> [_ w901]
        frame False {
        }
        frame True {
          n343 = for {
            tunnel: w903 -> [w914]
            tunnel: w904 -> [w913] mode=indexing
            tunnel: [w912] -> w902
            tunnel: w901 -> [w911]
            i -> [w910]
            n344 = case shown="\"Galil\"" w914 {
              tunnel: w910 -> [_ w920 w925 w931 _]
              tunnel: w913 -> [_ w921 w926 w932 _]
              tunnel: [_ w918 w924 _ _] -> w912
              tunnel: w911 -> [_ w917 w928 w930 _]
              frame "MM3000" {
                # "Don't 2nd axis if 0 plane dist"
              }
              frame "NI 735x", Default {
                n345 = Unbundle By Name(w917) -> ("Motion Bd ID"=w916:u8)
                n346 = Increment(x=w920) -> (x+1=w915:i32)
                n347 = call "MoveMotor.vi"("Position Mode (Absolute)"=0, "Target Position (0)"=w921, "Axis or Vector Space"=w915, "Motion Bd ID"=w916) -> ("error out"=w918:errorcluster)  [unwired: 5 in, 2 out]
              }
              frame "Galil" {
                n348 = Unbundle By Name(w928) -> ("GL Ref Out"=w927:refnum<k7>)
                n349 = call "GL Set Operation Mode.vi"("position cts (abs/rel)"=w926, "Position Mode (Absolute)"=T18."Absolute Position", "Start Now?"=TRUE, "Axis"=w925, "Galil.IGalil"=w927) -> ("error out"=w924:errorcluster)  [unwired: 4 in, 2 out]
              }
              frame "Newport ESP" {
                # "Don't 2nd axis if 0 plane dist"
                n350 = Unbundle By Name(w930) -> ("ESP VISA"=w929:refnum<visa-resource-name>)
                n351 = call <instrlib>:"Move Absolute.vi"("Position (0 units)"=w932, "Axis (1)"=w931, "VISA resource name"=w929) -> ()  [unwired: 3 in, 2 out]
              }
              frame "No Motion Card" {
              }
            }
          }
          n352 = case shown="\"Newport ESP\"" w903 {
            tunnel: w902 -> [_ w907 _]
            tunnel: w901 -> [_ w906 _]
            frame "MM3000" {
            }
            frame "Newport ESP" {
              n353 = Unbundle By Name(w906) -> ("ESP VISA"=w905:refnum<visa-resource-name>)
              n354 = stacked-sequence {
                tunnel: [w909 _] -> _
                tunnel: w907 -> [_ _]
                tunnel: w905 -> [w908 _]
                frame #0 {
                  n355 = call "WaitStopEPS.vi"("VISA resource name"=w908) -> ("Stopped"=w909:bool)  [unwired: 2 in, 2 out]
                }
                frame #1 {
                }
              }
            }
            frame "NI 735x", Default {
            }
          }
        }
      }
    }
    frame #14 {
      # "Email finish of data acq"
      n356 = case shown="True" w937 {
        frame False {
        }
        frame True {
          # "Close Feedback window if 2D"
        }
      }
      n357 = Equal?(x="recipient", y="") -> (x = y?=w941:bool)
      n358 = Unbundle By Name(w936) -> ("Synth Foc?"=w935:bool)
      n359 = call "ClosePopUpWindow.vi"() -> ()  [unwired: 12 in]
      n360 = case shown="False" w941 {
        tunnel: "recipient" -> [w948 _]
        frame False {
          n361 = call <vilib>:"SMTP Email Send Message (Small).vi"("return address"="Satan@hell.com", "mail server"="nyro-domino01", "message"="Your data is now ready to eat.", "subject ([No Subject])"="Scan is finished", "recipient"=w948) -> ()  [unwired: 1 in, 6 out]
        }
        frame True {
        }
      }
      n362 = Bundle("File Name In"=w939, TRUE, "Synth Foc?"=w935, "Microscopy Scan Mode"="Microscopy Scan Mode") -> (→"Scan Params":T27)  [unwired: 1 out]
      n363 = call "StopScan.vi"("Close FP"=TRUE) -> ()  [unwired: 5 in, 1 out]
    }
    frame #15 {
      n364 = Unbundle By Name(w949) -> ("Data Ref RF"=w951:refnum<data-value>, "Data Ref Log"=w950:refnum<data-value>)
      n365 = Unbundle By Name(w949) -> ("Dig Config"=w952:T12)
      n366 = Delete Data Value Reference(data value reference=w950) -> ()  [unwired: 1 in, 2 out]
      n367 = case shown="\"5-CH pulser w/ ann array\"" w952 {
        tunnel: w953 -> [_ w956]
        frame "Single channel", Default {
        }
        frame "5-CH pulser w/ ann array" {
          n368 = for {
            tunnel: w956 -> [w957] mode=indexing
            n369 = call <vilib>:"DAQmx Stop Task.vi"("task/channels in"=w957) -> ()  [unwired: 13 in, 2 out]
          }
        }
      }
      n370 = Delete Data Value Reference(data value reference=w951) -> ()  [unwired: 1 in, 2 out]
      n371 = case shown="3" w955 {
        tunnel: w954 -> [_ _ w958 w959]
        frame 0, Default {
        }
        frame 5 {
        }
        frame 3 {
          n372 = call <vilib>:"DAQmx Clear Task.vi"("task in"=w958) -> ()  [unwired: 1 in, 14 out]
        }
        frame 4 {
          n373 = call <vilib>:"DAQmx Clear Task.vi"("task in"=w959) -> ()  [unwired: 1 in, 14 out]
        }
      }
    }
    frame #16 {
      n374 = Unbundle By Name(w961) -> ("Motion System"=w962:T7)
      n375 = case shown="\"No Motion Card\", Default" w962 {
        tunnel: w961 -> [_ w964]
        tunnel: w960 -> [_ w963]
        frame "No Motion Card", Default {
        }
        frame "Galil" {
          n376 = case shown="True" w963 {
            tunnel: w964 -> [_ w968]
            frame False {
            }
            frame True {
              # "Use bit zero for turning on AND gate"
              n377 = Unbundle By Name(w968) -> ("GL Ref Out"=w966:refnum<k7>)
              n378 = for {
                N: 4 -> [_]
                shift-right: [w971] -> _
                shift-left: w966 -> [w975]
                tunnel: Command_Menu."Motor Off" ("Command") -> [w974]
                tunnel: [w969] -> _ mode=indexing
                i -> [w970]
                n379 = call "GL CheckForMotion.vi"("Axis"=w970, "Refnum in"=w975) -> ("Axis out"=w972:T19, "Refnum out"=w973:refnum<k7>)  [unwired: 7 in, 1 out]
                n380 = call "GL Command Set.vi"("Command"=w974, "Axis"=w972, "Galil.IGalil"=w973) -> ("error out"=w969:errorcluster, "ref out"=w971:refnum<k7>)  [unwired: 4 in, 3 out]
              }
            }
          }
        }
      }
    }
  }
  n381 = Or Array Elements(Boolean array=w37) -> (logical OR=w49:bool)
  n382 = Or Array Elements(Boolean array=w43) -> (logical OR=w46:bool)
  n383 = Unbundle(w34) -> ("source"=w33:string)  [unwired: 2 out]
  n384 = Subtract(x=w32, y=w31) -> (x-y=w30:u32)
  "x-y" <- w30
  n385 = Select(t="Motion Error.", s=w46, f="") -> (s? t:f=w40:string)
  n386 = Select(t=" Triggers Missing", s=w49, f="") -> (s? t:f=w42:string)
  n387 = global write "MotionGlobals.vi" "Acq Time (ms)"(w30) -> ()
  n388 = Concatenate Strings(w40, w33, w42) -> (→"Error Message":string)
